vi "Read SerDes GPIO Bank.vi"(0 "verify serdes id":bool=TRUE, 2 "serdes id":T1=enum."SI 0 Deserializer") -> (4 "gpio bank input":T2, 6 "serdes id valid":bool)   [LabVIEW 2023, in "GettingStarted_Common_148X_FPGA.lvlib"]
uses:
  GettingStarted_Common_148X_FPGA.lvlib
  <instrlib>/FlexRIO/CSI-2/v2/FPGA/Types/GPIO Bank.ctl
  Types/SerDes Identifier.ctl
  <instrlib>/_niInstr/Basic Elements/v1/FPGA/niInstr Basic Elements v1 FPGA.lvlib
  <vilib>/eio/EIONode/EIONode.xnode
  <vilib>/rvi/eio/common/nirviEmuTemplateMethod_errors.vi
  <instrlib>/FlexRIO/CSI-2/v2/FPGA/NI CSI-2 API FPGA v2.lvlib
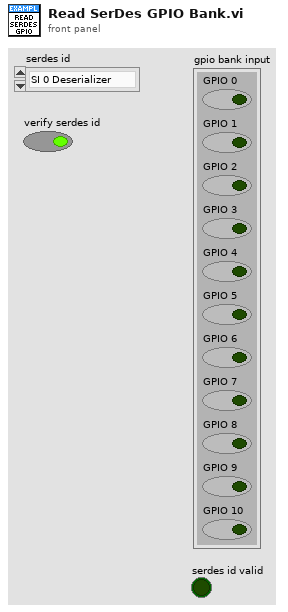
[diagram p1: front panel]
types:
  T1 = typedef "GettingStarted_Common_148X_FPGA.lvlib/SerDes Identifier.ctl" = enum8{"None", "SI 0 Deserializer", "SI 1 Deserializer", "SI 2 Deserializer", "SI 3 Deserializer", "SI 4 Deserializer", "SI 5 Deserializer", "SI 6 Deserializer", "SI 7 Deserializer", "SO 0 Serializer", "SO 1 Serializer", "SO 2 Serializer", "SO 3 Serializer", "SO 4 Serializer", "SO 5 Serializer", "SO 6 Serializer", "SO 7 Serializer", "SI 0 SI 1 Deserializer", "SI 2 SI 3 Deserializer", "SI 4 SI 5 Deserializer", "SI 6 SI 7 Deserializer"}
  T2 = typedef "NI CSI-2 API FPGA v2.lvlib/GPIO Bank.ctl" = cluster{"GPIO 0":bool, "GPIO 1":bool, "GPIO 2":bool, "GPIO 3":bool, "GPIO 4":bool, "GPIO 5":bool, "GPIO 6":bool, "GPIO 7":bool, "GPIO 8":bool, "GPIO 9":bool, "GPIO 10":bool}
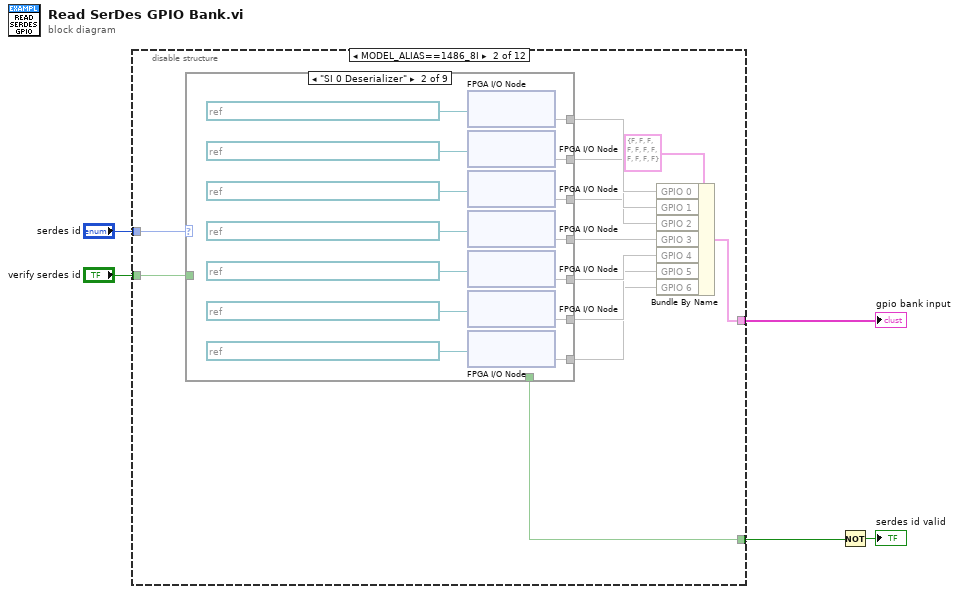
[diagram p0: block diagram]
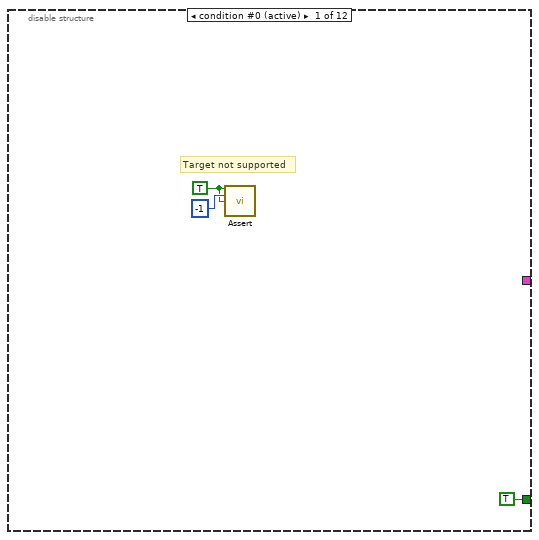
[diagram p2: hidden frame]
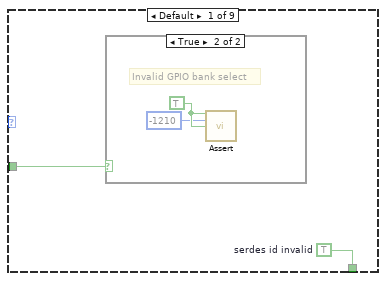
[diagram p3: hidden frame]
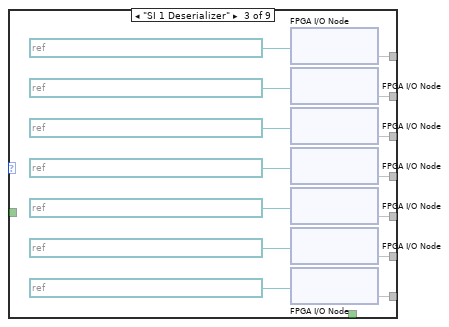
[diagram p5: hidden frame]
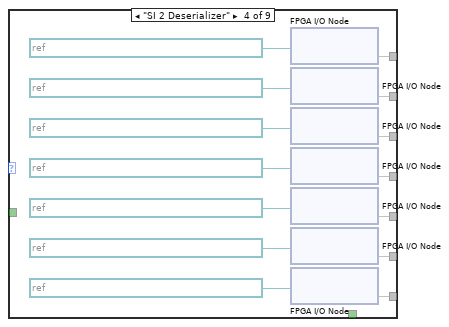
[diagram p6: hidden frame]
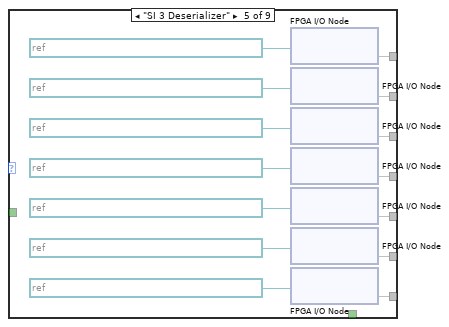
[diagram p7: hidden frame]
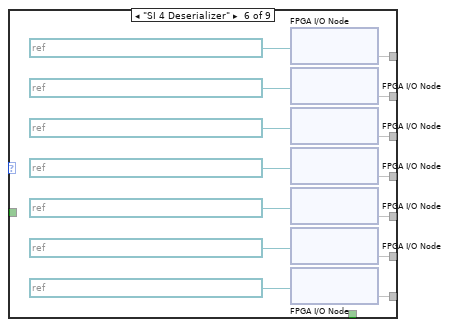
[diagram p8: hidden frame]
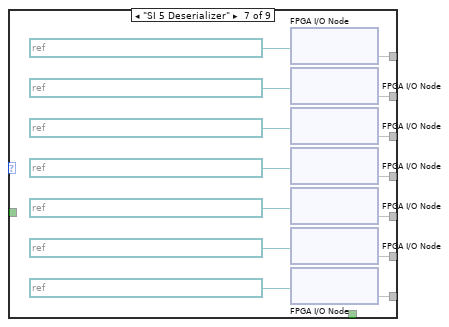
[diagram p9: hidden frame]
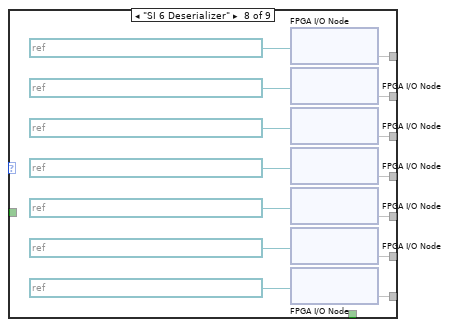
[diagram p10: hidden frame]
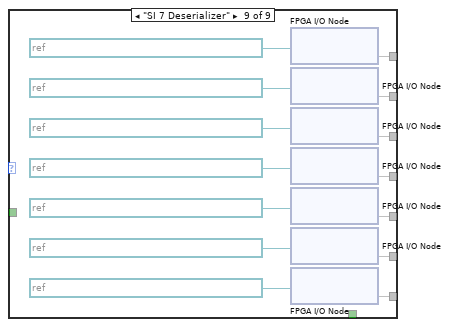
[diagram p11: hidden frame]
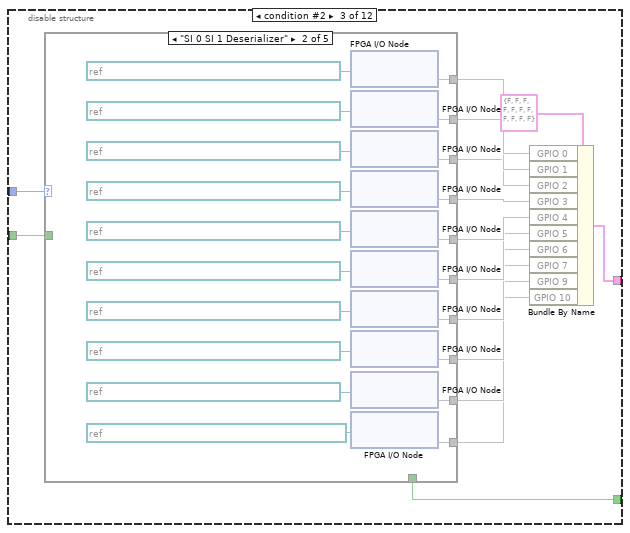
[diagram p12: hidden frame]
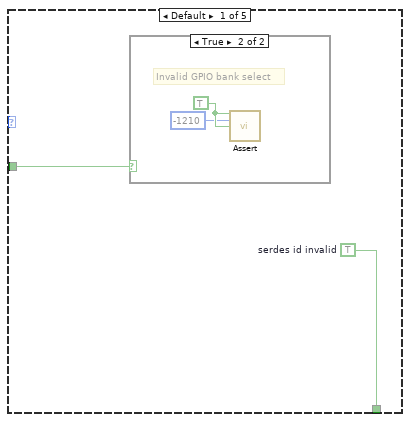
[diagram p13: hidden frame]
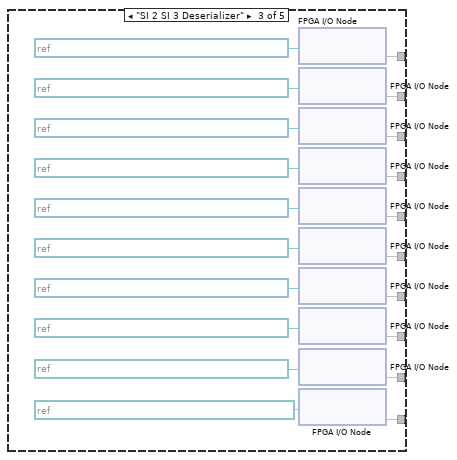
[diagram p15: hidden frame]
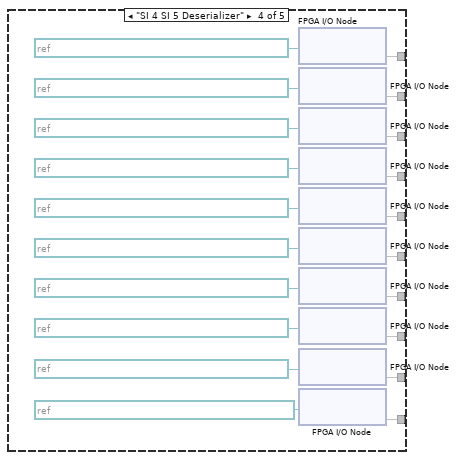
[diagram p16: hidden frame]
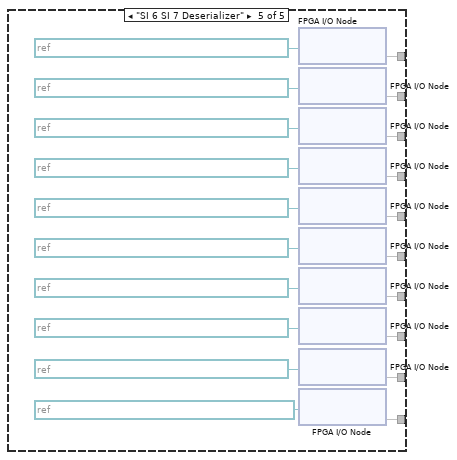
[diagram p17: hidden frame]
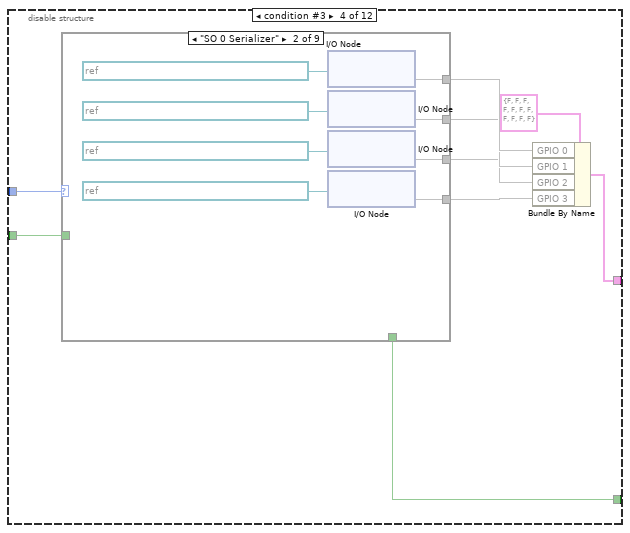
[diagram p18: hidden frame]
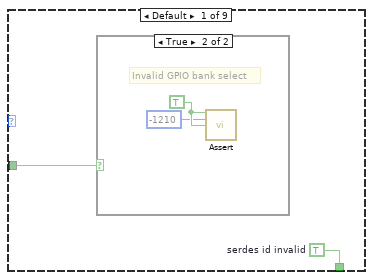
[diagram p19: hidden frame]
diagram:
  n1 = disable-structure shown="MODEL_ALIAS==1486_8I" {
    disable-tunnel: [_ w12 w143 w239 w316 w423 w556 w664 w725 w870 w953 w1125] -> w5
    disable-tunnel: "serdes id" -> [_ w11 w142 w238 w315 w422 w555 w663 w724 w869 w952 w1124]
    disable-tunnel: "verify serdes id" -> [_ w10 w141 w237 w314 w421 w549 w657 w721 w866 w949 w1121]
    disable-tunnel: [TRUE ("serdes gpio bank input select valid") w9 w140 w236 w313 w420 w548 w656 w720 w865 w948 w1120] -> w2
    frame condition #0 (active) {
      w7 = TRUE ("assert")
      # "Target not supported"
      n2 = call <instrlib>:"Assert.vi"("assert"=w7, "error code"=-1, "enable show error"=w7) -> ()  [unwired: 13 in]
    }
    frame condition #1 {
      n3 = case shown="\"SI 0 Deserializer\"" w11 {
        tunnel: [_ w32 w46 w60 w74 w88 w102 w116 w130] -> w19
        tunnel: [_ w31 w45 w59 w73 w87 w101 w115 w129] -> w18
        tunnel: [_ w30 w44 w58 w72 w86 w100 w114 w128] -> w17
        tunnel: [_ w29 w43 w57 w71 w85 w99 w113 w127] -> w16
        tunnel: [_ w28 w42 w56 w70 w84 w98 w112 w126] -> w15
        tunnel: [_ w27 w41 w55 w69 w83 w97 w111 w125] -> w14
        tunnel: [_ w25 w39 w53 w67 w81 w95 w109 w123] -> w13
        tunnel: w10 -> [w22 _ _ _ _ _ _ _ _]
        tunnel: [w21 _ _ _ _ _ _ _ _] -> w9
        frame Default {
          w21 = TRUE  # serdes id invalid
          n4 = case shown="True" w22 {
            frame False {
            }
            frame True {
              w24 = TRUE ("enable show error")
              # "Invalid GPIO bank select"
              n5 = call <instrlib>:"Assert.vi"("assert"=w24, "error code"=-1210, "enable show error"=w24) -> ()  [unwired: 13 in]
            }
          }
        }
        frame "SI 0 Deserializer" {
          n6 = xnode "FPGA I/O Node"("FPGA I/O In"=refnum<k21> "IO Socket\\SI 0 Deserializer GPIO 0 Input") -> ("I/O Item"=w32)  [unwired: 1 out]
          n7 = xnode "FPGA I/O Node"("FPGA I/O In"=refnum<k21> "IO Socket\\SI 0 Deserializer GPIO 1 Input") -> ("I/O Item"=w31)  [unwired: 1 out]
          n8 = xnode "FPGA I/O Node"("FPGA I/O In"=refnum<k21> "IO Socket\\SI 0 Deserializer GPIO 2 Input") -> ("I/O Item"=w30)  [unwired: 1 out]
          n9 = xnode "FPGA I/O Node"("FPGA I/O In"=refnum<k21> "IO Socket\\SI 0 Deserializer GPIO 3 Input") -> ("I/O Item"=w29)  [unwired: 1 out]
          n10 = xnode "FPGA I/O Node"("FPGA I/O In"=refnum<k21> "IO Socket\\SI 0 Deserializer GPIO 4 Input") -> ("I/O Item"=w28)  [unwired: 1 out]
          n11 = xnode "FPGA I/O Node"("FPGA I/O In"=refnum<k21> "IO Socket\\SI 0 Deserializer GPIO 5 Input") -> ("I/O Item"=w27)  [unwired: 1 out]
          n12 = xnode "FPGA I/O Node"("FPGA I/O In"=refnum<k21> "IO Socket\\SI 0 Deserializer GPIO 6 Input") -> ("I/O Item"=w25)  [unwired: 1 out]
        }
        frame "SI 1 Deserializer" {
          n13 = xnode "FPGA I/O Node"("FPGA I/O In"=refnum<k21> "IO Socket\\SI 1 Deserializer GPIO 0 Input") -> ("I/O Item"=w46)  [unwired: 1 out]
          n14 = xnode "FPGA I/O Node"("FPGA I/O In"=refnum<k21> "IO Socket\\SI 1 Deserializer GPIO 1 Input") -> ("I/O Item"=w45)  [unwired: 1 out]
          n15 = xnode "FPGA I/O Node"("FPGA I/O In"=refnum<k21> "IO Socket\\SI 1 Deserializer GPIO 2 Input") -> ("I/O Item"=w44)  [unwired: 1 out]
          n16 = xnode "FPGA I/O Node"("FPGA I/O In"=refnum<k21> "IO Socket\\SI 1 Deserializer GPIO 3 Input") -> ("I/O Item"=w43)  [unwired: 1 out]
          n17 = xnode "FPGA I/O Node"("FPGA I/O In"=refnum<k21> "IO Socket\\SI 1 Deserializer GPIO 4 Input") -> ("I/O Item"=w42)  [unwired: 1 out]
          n18 = xnode "FPGA I/O Node"("FPGA I/O In"=refnum<k21> "IO Socket\\SI 1 Deserializer GPIO 5 Input") -> ("I/O Item"=w41)  [unwired: 1 out]
          n19 = xnode "FPGA I/O Node"("FPGA I/O In"=refnum<k21> "IO Socket\\SI 1 Deserializer GPIO 6 Input") -> ("I/O Item"=w39)  [unwired: 1 out]
        }
        frame "SI 2 Deserializer" {
          n20 = xnode "FPGA I/O Node"("FPGA I/O In"=refnum<k21> "IO Socket\\SI 2 Deserializer GPIO 0 Input") -> ("I/O Item"=w60)  [unwired: 1 out]
          n21 = xnode "FPGA I/O Node"("FPGA I/O In"=refnum<k21> "IO Socket\\SI 2 Deserializer GPIO 1 Input") -> ("I/O Item"=w59)  [unwired: 1 out]
          n22 = xnode "FPGA I/O Node"("FPGA I/O In"=refnum<k21> "IO Socket\\SI 2 Deserializer GPIO 2 Input") -> ("I/O Item"=w58)  [unwired: 1 out]
          n23 = xnode "FPGA I/O Node"("FPGA I/O In"=refnum<k21> "IO Socket\\SI 2 Deserializer GPIO 3 Input") -> ("I/O Item"=w57)  [unwired: 1 out]
          n24 = xnode "FPGA I/O Node"("FPGA I/O In"=refnum<k21> "IO Socket\\SI 2 Deserializer GPIO 4 Input") -> ("I/O Item"=w56)  [unwired: 1 out]
          n25 = xnode "FPGA I/O Node"("FPGA I/O In"=refnum<k21> "IO Socket\\SI 2 Deserializer GPIO 5 Input") -> ("I/O Item"=w55)  [unwired: 1 out]
          n26 = xnode "FPGA I/O Node"("FPGA I/O In"=refnum<k21> "IO Socket\\SI 2 Deserializer GPIO 6 Input") -> ("I/O Item"=w53)  [unwired: 1 out]
        }
        frame "SI 3 Deserializer" {
          n27 = xnode "FPGA I/O Node"("FPGA I/O In"=refnum<k21> "IO Socket\\SI 3 Deserializer GPIO 0 Input") -> ("I/O Item"=w74)  [unwired: 1 out]
          n28 = xnode "FPGA I/O Node"("FPGA I/O In"=refnum<k21> "IO Socket\\SI 3 Deserializer GPIO 1 Input") -> ("I/O Item"=w73)  [unwired: 1 out]
          n29 = xnode "FPGA I/O Node"("FPGA I/O In"=refnum<k21> "IO Socket\\SI 3 Deserializer GPIO 2 Input") -> ("I/O Item"=w72)  [unwired: 1 out]
          n30 = xnode "FPGA I/O Node"("FPGA I/O In"=refnum<k21> "IO Socket\\SI 3 Deserializer GPIO 3 Input") -> ("I/O Item"=w71)  [unwired: 1 out]
          n31 = xnode "FPGA I/O Node"("FPGA I/O In"=refnum<k21> "IO Socket\\SI 3 Deserializer GPIO 4 Input") -> ("I/O Item"=w70)  [unwired: 1 out]
          n32 = xnode "FPGA I/O Node"("FPGA I/O In"=refnum<k21> "IO Socket\\SI 3 Deserializer GPIO 5 Input") -> ("I/O Item"=w69)  [unwired: 1 out]
          n33 = xnode "FPGA I/O Node"("FPGA I/O In"=refnum<k21> "IO Socket\\SI 3 Deserializer GPIO 6 Input") -> ("I/O Item"=w67)  [unwired: 1 out]
        }
        frame "SI 4 Deserializer" {
          n34 = xnode "FPGA I/O Node"("FPGA I/O In"=refnum<k21> "IO Socket\\SI 4 Deserializer GPIO 0 Input") -> ("I/O Item"=w88)  [unwired: 1 out]
          n35 = xnode "FPGA I/O Node"("FPGA I/O In"=refnum<k21> "IO Socket\\SI 4 Deserializer GPIO 1 Input") -> ("I/O Item"=w87)  [unwired: 1 out]
          n36 = xnode "FPGA I/O Node"("FPGA I/O In"=refnum<k21> "IO Socket\\SI 4 Deserializer GPIO 2 Input") -> ("I/O Item"=w86)  [unwired: 1 out]
          n37 = xnode "FPGA I/O Node"("FPGA I/O In"=refnum<k21> "IO Socket\\SI 4 Deserializer GPIO 3 Input") -> ("I/O Item"=w85)  [unwired: 1 out]
          n38 = xnode "FPGA I/O Node"("FPGA I/O In"=refnum<k21> "IO Socket\\SI 4 Deserializer GPIO 4 Input") -> ("I/O Item"=w84)  [unwired: 1 out]
          n39 = xnode "FPGA I/O Node"("FPGA I/O In"=refnum<k21> "IO Socket\\SI 4 Deserializer GPIO 5 Input") -> ("I/O Item"=w83)  [unwired: 1 out]
          n40 = xnode "FPGA I/O Node"("FPGA I/O In"=refnum<k21> "IO Socket\\SI 4 Deserializer GPIO 6 Input") -> ("I/O Item"=w81)  [unwired: 1 out]
        }
        frame "SI 5 Deserializer" {
          n41 = xnode "FPGA I/O Node"("FPGA I/O In"=refnum<k21> "IO Socket\\SI 5 Deserializer GPIO 0 Input") -> ("I/O Item"=w102)  [unwired: 1 out]
          n42 = xnode "FPGA I/O Node"("FPGA I/O In"=refnum<k21> "IO Socket\\SI 5 Deserializer GPIO 1 Input") -> ("I/O Item"=w101)  [unwired: 1 out]
          n43 = xnode "FPGA I/O Node"("FPGA I/O In"=refnum<k21> "IO Socket\\SI 5 Deserializer GPIO 2 Input") -> ("I/O Item"=w100)  [unwired: 1 out]
          n44 = xnode "FPGA I/O Node"("FPGA I/O In"=refnum<k21> "IO Socket\\SI 5 Deserializer GPIO 3 Input") -> ("I/O Item"=w99)  [unwired: 1 out]
          n45 = xnode "FPGA I/O Node"("FPGA I/O In"=refnum<k21> "IO Socket\\SI 5 Deserializer GPIO 4 Input") -> ("I/O Item"=w98)  [unwired: 1 out]
          n46 = xnode "FPGA I/O Node"("FPGA I/O In"=refnum<k21> "IO Socket\\SI 5 Deserializer GPIO 5 Input") -> ("I/O Item"=w97)  [unwired: 1 out]
          n47 = xnode "FPGA I/O Node"("FPGA I/O In"=refnum<k21> "IO Socket\\SI 5 Deserializer GPIO 6 Input") -> ("I/O Item"=w95)  [unwired: 1 out]
        }
        frame "SI 6 Deserializer" {
          n48 = xnode "FPGA I/O Node"("FPGA I/O In"=refnum<k21> "IO Socket\\SI 6 Deserializer GPIO 0 Input") -> ("I/O Item"=w116)  [unwired: 1 out]
          n49 = xnode "FPGA I/O Node"("FPGA I/O In"=refnum<k21> "IO Socket\\SI 6 Deserializer GPIO 1 Input") -> ("I/O Item"=w115)  [unwired: 1 out]
          n50 = xnode "FPGA I/O Node"("FPGA I/O In"=refnum<k21> "IO Socket\\SI 6 Deserializer GPIO 2 Input") -> ("I/O Item"=w114)  [unwired: 1 out]
          n51 = xnode "FPGA I/O Node"("FPGA I/O In"=refnum<k21> "IO Socket\\SI 6 Deserializer GPIO 3 Input") -> ("I/O Item"=w113)  [unwired: 1 out]
          n52 = xnode "FPGA I/O Node"("FPGA I/O In"=refnum<k21> "IO Socket\\SI 6 Deserializer GPIO 4 Input") -> ("I/O Item"=w112)  [unwired: 1 out]
          n53 = xnode "FPGA I/O Node"("FPGA I/O In"=refnum<k21> "IO Socket\\SI 6 Deserializer GPIO 5 Input") -> ("I/O Item"=w111)  [unwired: 1 out]
          n54 = xnode "FPGA I/O Node"("FPGA I/O In"=refnum<k21> "IO Socket\\SI 6 Deserializer GPIO 6 Input") -> ("I/O Item"=w109)  [unwired: 1 out]
        }
        frame "SI 7 Deserializer" {
          n55 = xnode "FPGA I/O Node"("FPGA I/O In"=refnum<k21> "IO Socket\\SI 7 Deserializer GPIO 0 Input") -> ("I/O Item"=w130)  [unwired: 1 out]
          n56 = xnode "FPGA I/O Node"("FPGA I/O In"=refnum<k21> "IO Socket\\SI 7 Deserializer GPIO 1 Input") -> ("I/O Item"=w129)  [unwired: 1 out]
          n57 = xnode "FPGA I/O Node"("FPGA I/O In"=refnum<k21> "IO Socket\\SI 7 Deserializer GPIO 2 Input") -> ("I/O Item"=w128)  [unwired: 1 out]
          n58 = xnode "FPGA I/O Node"("FPGA I/O In"=refnum<k21> "IO Socket\\SI 7 Deserializer GPIO 3 Input") -> ("I/O Item"=w127)  [unwired: 1 out]
          n59 = xnode "FPGA I/O Node"("FPGA I/O In"=refnum<k21> "IO Socket\\SI 7 Deserializer GPIO 4 Input") -> ("I/O Item"=w126)  [unwired: 1 out]
          n60 = xnode "FPGA I/O Node"("FPGA I/O In"=refnum<k21> "IO Socket\\SI 7 Deserializer GPIO 5 Input") -> ("I/O Item"=w125)  [unwired: 1 out]
          n61 = xnode "FPGA I/O Node"("FPGA I/O In"=refnum<k21> "IO Socket\\SI 7 Deserializer GPIO 6 Input") -> ("I/O Item"=w123)  [unwired: 1 out]
        }
      }
      n62 = Bundle By Name(cluster=T2 {"GPIO 0"=FALSE, "GPIO 1"=FALSE, "GPIO 2"=FALSE, "GPIO 3"=FALSE, "GPIO 4"=FALSE, "GPIO 5"=FALSE, "GPIO 6"=FALSE, "GPIO 7"=FALSE, "GPIO 8"=FALSE, "GPIO 9"=FALSE, "GPIO 10"=FALSE} ("gpio bank"), "GPIO 0"=w19, "GPIO 1"=w18, "GPIO 2"=w17, "GPIO 3"=w16, "GPIO 4"=w15, "GPIO 5"=w14, "GPIO 6"=w13) -> (w12:T2)
    }
    frame condition #2 {
      n63 = case shown="\"SI 0 SI 1 Deserializer\"" w142 {
        tunnel: [_ w173 w193 w213 w233] -> w150
        tunnel: [_ w172 w192 w212 w232] -> w149
        tunnel: [_ w171 w191 w211 w231] -> w148
        tunnel: [_ w170 w190 w210 w230] -> w147
        tunnel: [_ w169 w189 w209 w229] -> w146
        tunnel: [_ w168 w188 w208 w228] -> w145
        tunnel: [_ w167 w187 w207 w227] -> w144
        tunnel: w141 -> [w153 _ _ _ _]
        tunnel: [w152 _ _ _ _] -> w140
        tunnel: [_ w165 w185 w205 w225] -> w139
        tunnel: [_ w156 w176 w196 w216] -> w138
        tunnel: [_ w157 w177 w197 w217] -> w137
        frame Default {
          w152 = TRUE  # serdes id invalid
          n64 = case shown="True" w153 {
            frame False {
            }
            frame True {
              w155 = TRUE ("enable show error")
              # "Invalid GPIO bank select"
              n65 = call <instrlib>:"Assert.vi"("assert"=w155, "error code"=-1210, "enable show error"=w155) -> ()  [unwired: 13 in]
            }
          }
        }
        frame "SI 0 SI 1 Deserializer" {
          n66 = xnode "FPGA I/O Node"("FPGA I/O In"=refnum<k21> "IO Socket\\SI 0 SI 1 Deserializer GPIO 0 Input") -> ("I/O Item"=w173)  [unwired: 1 out]
          n67 = xnode "FPGA I/O Node"("FPGA I/O In"=refnum<k21> "IO Socket\\SI 0 SI 1 Deserializer GPIO 1 Input") -> ("I/O Item"=w172)  [unwired: 1 out]
          n68 = xnode "FPGA I/O Node"("FPGA I/O In"=refnum<k21> "IO Socket\\SI 0 SI 1 Deserializer GPIO 2 Input") -> ("I/O Item"=w171)  [unwired: 1 out]
          n69 = xnode "FPGA I/O Node"("FPGA I/O In"=refnum<k21> "IO Socket\\SI 0 SI 1 Deserializer GPIO 3 Input") -> ("I/O Item"=w170)  [unwired: 1 out]
          n70 = xnode "FPGA I/O Node"("FPGA I/O In"=refnum<k21> "IO Socket\\SI 0 SI 1 Deserializer GPIO 4 Input") -> ("I/O Item"=w169)  [unwired: 1 out]
          n71 = xnode "FPGA I/O Node"("FPGA I/O In"=refnum<k21> "IO Socket\\SI 0 SI 1 Deserializer GPIO 5 Input") -> ("I/O Item"=w168)  [unwired: 1 out]
          n72 = xnode "FPGA I/O Node"("FPGA I/O In"=refnum<k21> "IO Socket\\SI 0 SI 1 Deserializer GPIO 6 Input") -> ("I/O Item"=w167)  [unwired: 1 out]
          n73 = xnode "FPGA I/O Node"("FPGA I/O In"=refnum<k21> "IO Socket\\SI 0 SI 1 Deserializer GPIO 7 Input") -> ("I/O Item"=w165)  [unwired: 1 out]
          n74 = xnode "FPGA I/O Node"("FPGA I/O In"=refnum<k21> "IO Socket\\SI 0 SI 1 Deserializer GPIO 9 Input") -> ("I/O Item"=w156)  [unwired: 1 out]
          n75 = xnode "FPGA I/O Node"("FPGA I/O In"=refnum<k21> "IO Socket\\SI 0 SI 1 Deserializer GPIO 10 Input") -> ("I/O Item"=w157)  [unwired: 1 out]
        }
        frame "SI 2 SI 3 Deserializer" {
          n76 = xnode "FPGA I/O Node"("FPGA I/O In"=refnum<k21> "IO Socket\\SI 2 SI 3 Deserializer GPIO 0 Input") -> ("I/O Item"=w193)  [unwired: 1 out]
          n77 = xnode "FPGA I/O Node"("FPGA I/O In"=refnum<k21> "IO Socket\\SI 2 SI 3 Deserializer GPIO 1 Input") -> ("I/O Item"=w192)  [unwired: 1 out]
          n78 = xnode "FPGA I/O Node"("FPGA I/O In"=refnum<k21> "IO Socket\\SI 2 SI 3 Deserializer GPIO 2 Input") -> ("I/O Item"=w191)  [unwired: 1 out]
          n79 = xnode "FPGA I/O Node"("FPGA I/O In"=refnum<k21> "IO Socket\\SI 2 SI 3 Deserializer GPIO 3 Input") -> ("I/O Item"=w190)  [unwired: 1 out]
          n80 = xnode "FPGA I/O Node"("FPGA I/O In"=refnum<k21> "IO Socket\\SI 2 SI 3 Deserializer GPIO 4 Input") -> ("I/O Item"=w189)  [unwired: 1 out]
          n81 = xnode "FPGA I/O Node"("FPGA I/O In"=refnum<k21> "IO Socket\\SI 2 SI 3 Deserializer GPIO 5 Input") -> ("I/O Item"=w188)  [unwired: 1 out]
          n82 = xnode "FPGA I/O Node"("FPGA I/O In"=refnum<k21> "IO Socket\\SI 2 SI 3 Deserializer GPIO 6 Input") -> ("I/O Item"=w187)  [unwired: 1 out]
          n83 = xnode "FPGA I/O Node"("FPGA I/O In"=refnum<k21> "IO Socket\\SI 2 SI 3 Deserializer GPIO 7 Input") -> ("I/O Item"=w185)  [unwired: 1 out]
          n84 = xnode "FPGA I/O Node"("FPGA I/O In"=refnum<k21> "IO Socket\\SI 2 SI 3 Deserializer GPIO 9 Input") -> ("I/O Item"=w176)  [unwired: 1 out]
          n85 = xnode "FPGA I/O Node"("FPGA I/O In"=refnum<k21> "IO Socket\\SI 2 SI 3 Deserializer GPIO 10 Input") -> ("I/O Item"=w177)  [unwired: 1 out]
        }
        frame "SI 4 SI 5 Deserializer" {
          n86 = xnode "FPGA I/O Node"("FPGA I/O In"=refnum<k21> "IO Socket\\SI 4 SI 5 Deserializer GPIO 0 Input") -> ("I/O Item"=w213)  [unwired: 1 out]
          n87 = xnode "FPGA I/O Node"("FPGA I/O In"=refnum<k21> "IO Socket\\SI 4 SI 5 Deserializer GPIO 1 Input") -> ("I/O Item"=w212)  [unwired: 1 out]
          n88 = xnode "FPGA I/O Node"("FPGA I/O In"=refnum<k21> "IO Socket\\SI 4 SI 5 Deserializer GPIO 2 Input") -> ("I/O Item"=w211)  [unwired: 1 out]
          n89 = xnode "FPGA I/O Node"("FPGA I/O In"=refnum<k21> "IO Socket\\SI 4 SI 5 Deserializer GPIO 3 Input") -> ("I/O Item"=w210)  [unwired: 1 out]
          n90 = xnode "FPGA I/O Node"("FPGA I/O In"=refnum<k21> "IO Socket\\SI 4 SI 5 Deserializer GPIO 4 Input") -> ("I/O Item"=w209)  [unwired: 1 out]
          n91 = xnode "FPGA I/O Node"("FPGA I/O In"=refnum<k21> "IO Socket\\SI 4 SI 5 Deserializer GPIO 5 Input") -> ("I/O Item"=w208)  [unwired: 1 out]
          n92 = xnode "FPGA I/O Node"("FPGA I/O In"=refnum<k21> "IO Socket\\SI 4 SI 5 Deserializer GPIO 6 Input") -> ("I/O Item"=w207)  [unwired: 1 out]
          n93 = xnode "FPGA I/O Node"("FPGA I/O In"=refnum<k21> "IO Socket\\SI 4 SI 5 Deserializer GPIO 7 Input") -> ("I/O Item"=w205)  [unwired: 1 out]
          n94 = xnode "FPGA I/O Node"("FPGA I/O In"=refnum<k21> "IO Socket\\SI 4 SI 5 Deserializer GPIO 9 Input") -> ("I/O Item"=w196)  [unwired: 1 out]
          n95 = xnode "FPGA I/O Node"("FPGA I/O In"=refnum<k21> "IO Socket\\SI 4 SI 5 Deserializer GPIO 10 Input") -> ("I/O Item"=w197)  [unwired: 1 out]
        }
        frame "SI 6 SI 7 Deserializer" {
          n96 = xnode "FPGA I/O Node"("FPGA I/O In"=refnum<k21> "IO Socket\\SI 6 SI 7 Deserializer GPIO 0 Input") -> ("I/O Item"=w233)  [unwired: 1 out]
          n97 = xnode "FPGA I/O Node"("FPGA I/O In"=refnum<k21> "IO Socket\\SI 6 SI 7 Deserializer GPIO 1 Input") -> ("I/O Item"=w232)  [unwired: 1 out]
          n98 = xnode "FPGA I/O Node"("FPGA I/O In"=refnum<k21> "IO Socket\\SI 6 SI 7 Deserializer GPIO 2 Input") -> ("I/O Item"=w231)  [unwired: 1 out]
          n99 = xnode "FPGA I/O Node"("FPGA I/O In"=refnum<k21> "IO Socket\\SI 6 SI 7 Deserializer GPIO 3 Input") -> ("I/O Item"=w230)  [unwired: 1 out]
          n100 = xnode "FPGA I/O Node"("FPGA I/O In"=refnum<k21> "IO Socket\\SI 6 SI 7 Deserializer GPIO 4 Input") -> ("I/O Item"=w229)  [unwired: 1 out]
          n101 = xnode "FPGA I/O Node"("FPGA I/O In"=refnum<k21> "IO Socket\\SI 6 SI 7 Deserializer GPIO 5 Input") -> ("I/O Item"=w228)  [unwired: 1 out]
          n102 = xnode "FPGA I/O Node"("FPGA I/O In"=refnum<k21> "IO Socket\\SI 6 SI 7 Deserializer GPIO 6 Input") -> ("I/O Item"=w227)  [unwired: 1 out]
          n103 = xnode "FPGA I/O Node"("FPGA I/O In"=refnum<k21> "IO Socket\\SI 6 SI 7 Deserializer GPIO 7 Input") -> ("I/O Item"=w225)  [unwired: 1 out]
          n104 = xnode "FPGA I/O Node"("FPGA I/O In"=refnum<k21> "IO Socket\\SI 6 SI 7 Deserializer GPIO 9 Input") -> ("I/O Item"=w216)  [unwired: 1 out]
          n105 = xnode "FPGA I/O Node"("FPGA I/O In"=refnum<k21> "IO Socket\\SI 6 SI 7 Deserializer GPIO 10 Input") -> ("I/O Item"=w217)  [unwired: 1 out]
        }
      }
      n106 = Bundle By Name(cluster=T2 {"GPIO 0"=FALSE, "GPIO 1"=FALSE, "GPIO 2"=FALSE, "GPIO 3"=FALSE, "GPIO 4"=FALSE, "GPIO 5"=FALSE, "GPIO 6"=FALSE, "GPIO 7"=FALSE, "GPIO 8"=FALSE, "GPIO 9"=FALSE, "GPIO 10"=FALSE} ("gpio bank"), "GPIO 0"=w150, "GPIO 1"=w149, "GPIO 2"=w148, "GPIO 3"=w147, "GPIO 4"=w146, "GPIO 5"=w145, "GPIO 6"=w144, "GPIO 7"=w139, "GPIO 9"=w138, "GPIO 10"=w137) -> (w143:T2)
    }
    frame condition #3 {
      n107 = case shown="\"SO 0 Serializer\"" w238 {
        tunnel: [_ w252 w260 w268 w276 w284 w292 w300 w308] -> w243
        tunnel: [_ w251 w259 w267 w275 w283 w291 w299 w307] -> w242
        tunnel: [_ w250 w258 w266 w274 w282 w290 w298 w306] -> w241
        tunnel: [_ w249 w257 w265 w273 w281 w289 w297 w305] -> w240
        tunnel: w237 -> [w246 _ _ _ _ _ _ _ _]
        tunnel: [w245 _ _ _ _ _ _ _ _] -> w236
        frame Default {
          w245 = TRUE  # serdes id invalid
          n108 = case shown="True" w246 {
            frame False {
            }
            frame True {
              w248 = TRUE ("enable show error")
              # "Invalid GPIO bank select"
              n109 = call <instrlib>:"Assert.vi"("assert"=w248, "error code"=-1210, "enable show error"=w248) -> ()  [unwired: 13 in]
            }
          }
        }
        frame "SO 0 Serializer" {
          n110 = xnode "I/O Node"("FPGA I/O In"=refnum<k21> "IO Socket\\SO 0 Serializer GPIO 0 Input") -> ("I/O Item"=w252)  [unwired: 1 out]
          n111 = xnode "I/O Node"("FPGA I/O In"=refnum<k21> "IO Socket\\SO 0 Serializer GPIO 1 Input") -> ("I/O Item"=w251)  [unwired: 1 out]
          n112 = xnode "I/O Node"("FPGA I/O In"=refnum<k21> "IO Socket\\SO 0 Serializer GPIO 2 Input") -> ("I/O Item"=w250)  [unwired: 1 out]
          n113 = xnode "I/O Node"("FPGA I/O In"=refnum<k21> "IO Socket\\SO 0 Serializer GPIO 3 Input") -> ("I/O Item"=w249)  [unwired: 1 out]
        }
        frame "SO 1 Serializer" {
          n114 = xnode "I/O Node"("FPGA I/O In"=refnum<k21> "IO Socket\\SO 1 Serializer GPIO 0 Input") -> ("I/O Item"=w260)  [unwired: 1 out]
          n115 = xnode "I/O Node"("FPGA I/O In"=refnum<k21> "IO Socket\\SO 1 Serializer GPIO 1 Input") -> ("I/O Item"=w259)  [unwired: 1 out]
          n116 = xnode "I/O Node"("FPGA I/O In"=refnum<k21> "IO Socket\\SO 1 Serializer GPIO 2 Input") -> ("I/O Item"=w258)  [unwired: 1 out]
          n117 = xnode "I/O Node"("FPGA I/O In"=refnum<k21> "IO Socket\\SO 1 Serializer GPIO 3 Input") -> ("I/O Item"=w257)  [unwired: 1 out]
        }
        frame "SO 2 Serializer" {
          n118 = xnode "I/O Node"("FPGA I/O In"=refnum<k21> "IO Socket\\SO 2 Serializer GPIO 0 Input") -> ("I/O Item"=w268)  [unwired: 1 out]
          n119 = xnode "I/O Node"("FPGA I/O In"=refnum<k21> "IO Socket\\SO 2 Serializer GPIO 1 Input") -> ("I/O Item"=w267)  [unwired: 1 out]
          n120 = xnode "I/O Node"("FPGA I/O In"=refnum<k21> "IO Socket\\SO 2 Serializer GPIO 2 Input") -> ("I/O Item"=w266)  [unwired: 1 out]
          n121 = xnode "I/O Node"("FPGA I/O In"=refnum<k21> "IO Socket\\SO 2 Serializer GPIO 3 Input") -> ("I/O Item"=w265)  [unwired: 1 out]
        }
        frame "SO 3 Serializer" {
          n122 = xnode "I/O Node"("FPGA I/O In"=refnum<k21> "IO Socket\\SO 3 Serializer GPIO 0 Input") -> ("I/O Item"=w276)  [unwired: 1 out]
          n123 = xnode "I/O Node"("FPGA I/O In"=refnum<k21> "IO Socket\\SO 3 Serializer GPIO 1 Input") -> ("I/O Item"=w275)  [unwired: 1 out]
          n124 = xnode "FPGA I/O Node"("FPGA I/O In"=refnum<k21> "IO Socket\\SO 3 Serializer GPIO 2 Input") -> ("I/O Item"=w274)  [unwired: 1 out]
          n125 = xnode "I/O Node"("FPGA I/O In"=refnum<k21> "IO Socket\\SO 3 Serializer GPIO 3 Input") -> ("I/O Item"=w273)  [unwired: 1 out]
        }
        frame "SO 4 Serializer" {
          n126 = xnode "I/O Node"("FPGA I/O In"=refnum<k21> "IO Socket\\SO 4 Serializer GPIO 0 Input") -> ("I/O Item"=w284)  [unwired: 1 out]
          n127 = xnode "I/O Node"("FPGA I/O In"=refnum<k21> "IO Socket\\SO 4 Serializer GPIO 1 Input") -> ("I/O Item"=w283)  [unwired: 1 out]
          n128 = xnode "I/O Node"("FPGA I/O In"=refnum<k21> "IO Socket\\SO 4 Serializer GPIO 2 Input") -> ("I/O Item"=w282)  [unwired: 1 out]
          n129 = xnode "I/O Node"("FPGA I/O In"=refnum<k21> "IO Socket\\SO 4 Serializer GPIO 3 Input") -> ("I/O Item"=w281)  [unwired: 1 out]
        }
        frame "SO 5 Serializer" {
          n130 = xnode "I/O Node"("FPGA I/O In"=refnum<k21> "IO Socket\\SO 5 Serializer GPIO 0 Input") -> ("I/O Item"=w292)  [unwired: 1 out]
          n131 = xnode "I/O Node"("FPGA I/O In"=refnum<k21> "IO Socket\\SO 5 Serializer GPIO 1 Input") -> ("I/O Item"=w291)  [unwired: 1 out]
          n132 = xnode "I/O Node"("FPGA I/O In"=refnum<k21> "IO Socket\\SO 5 Serializer GPIO 2 Input") -> ("I/O Item"=w290)  [unwired: 1 out]
          n133 = xnode "I/O Node"("FPGA I/O In"=refnum<k21> "IO Socket\\SO 5 Serializer GPIO 3 Input") -> ("I/O Item"=w289)  [unwired: 1 out]
        }
        frame "SO 6 Serializer" {
          n134 = xnode "I/O Node"("FPGA I/O In"=refnum<k21> "IO Socket\\SO 6 Serializer GPIO 0 Input") -> ("I/O Item"=w300)  [unwired: 1 out]
          n135 = xnode "I/O Node"("FPGA I/O In"=refnum<k21> "IO Socket\\SO 6 Serializer GPIO 1 Input") -> ("I/O Item"=w299)  [unwired: 1 out]
          n136 = xnode "I/O Node"("FPGA I/O In"=refnum<k21> "IO Socket\\SO 6 Serializer GPIO 2 Input") -> ("I/O Item"=w298)  [unwired: 1 out]
          n137 = xnode "I/O Node"("FPGA I/O In"=refnum<k21> "IO Socket\\SO 6 Serializer GPIO 3 Input") -> ("I/O Item"=w297)  [unwired: 1 out]
        }
        frame "SO 7 Serializer" {
          n138 = xnode "I/O Node"("FPGA I/O In"=refnum<k21> "IO Socket\\SO 7 Serializer GPIO 0 Input") -> ("I/O Item"=w308)  [unwired: 1 out]
          n139 = xnode "FPGA I/O Node"("FPGA I/O In"=refnum<k21> "IO Socket\\SO 7 Serializer GPIO 1 Input") -> ("I/O Item"=w307)  [unwired: 1 out]
          n140 = xnode "I/O Node"("FPGA I/O In"=refnum<k21> "IO Socket\\SO 7 Serializer GPIO 2 Input") -> ("I/O Item"=w306)  [unwired: 1 out]
          n141 = xnode "I/O Node"("FPGA I/O In"=refnum<k21> "IO Socket\\SO 7 Serializer GPIO 3 Input") -> ("I/O Item"=w305)  [unwired: 1 out]
        }
      }
      n142 = Bundle By Name(cluster=T2 {"GPIO 0"=FALSE, "GPIO 1"=FALSE, "GPIO 2"=FALSE, "GPIO 3"=FALSE, "GPIO 4"=FALSE, "GPIO 5"=FALSE, "GPIO 6"=FALSE, "GPIO 7"=FALSE, "GPIO 8"=FALSE, "GPIO 9"=FALSE, "GPIO 10"=FALSE} ("gpio bank"), "GPIO 0"=w243, "GPIO 1"=w242, "GPIO 2"=w241, "GPIO 3"=w240) -> (w239:T2)
    }
    frame condition #4 {
      n143 = case shown="\"SI 0 Deserializer\"" w315 {
        tunnel: [_ w336 w350 w364 w378 w388 w396 w404 w412] -> w323
        tunnel: [_ w335 w349 w363 w377 w387 w395 w403 w411] -> w322
        tunnel: [_ w334 w348 w362 w376 w386 w394 w402 w410] -> w321
        tunnel: [_ w333 w347 w361 w375 w385 w393 w401 w409] -> w320
        tunnel: [_ w332 w346 w360 w374 _ _ _ _] -> w319
        tunnel: [_ w331 w345 w359 w373 _ _ _ _] -> w318
        tunnel: [_ w329 w343 w357 w371 _ _ _ _] -> w317
        tunnel: w314 -> [w326 _ _ _ _ _ _ _ _]
        tunnel: [w325 _ _ _ _ _ _ _ _] -> w313
        frame Default {
          w325 = TRUE  # serdes id invalid
          n144 = case shown="True" w326 {
            frame False {
            }
            frame True {
              w328 = TRUE ("enable show error")
              # "Invalid GPIO bank select"
              n145 = call <instrlib>:"Assert.vi"("assert"=w328, "error code"=-1210, "enable show error"=w328) -> ()  [unwired: 13 in]
            }
          }
        }
        frame "SI 0 Deserializer" {
          n146 = xnode "FPGA I/O Node"("FPGA I/O In"=refnum<k21> "IO Socket\\SI 0 Deserializer GPIO 0 Input") -> ("I/O Item"=w336)  [unwired: 1 out]
          n147 = xnode "FPGA I/O Node"("FPGA I/O In"=refnum<k21> "IO Socket\\SI 0 Deserializer GPIO 1 Input") -> ("I/O Item"=w335)  [unwired: 1 out]
          n148 = xnode "FPGA I/O Node"("FPGA I/O In"=refnum<k21> "IO Socket\\SI 0 Deserializer GPIO 2 Input") -> ("I/O Item"=w334)  [unwired: 1 out]
          n149 = xnode "FPGA I/O Node"("FPGA I/O In"=refnum<k21> "IO Socket\\SI 0 Deserializer GPIO 3 Input") -> ("I/O Item"=w333)  [unwired: 1 out]
          n150 = xnode "FPGA I/O Node"("FPGA I/O In"=refnum<k21> "IO Socket\\SI 0 Deserializer GPIO 4 Input") -> ("I/O Item"=w332)  [unwired: 1 out]
          n151 = xnode "FPGA I/O Node"("FPGA I/O In"=refnum<k21> "IO Socket\\SI 0 Deserializer GPIO 5 Input") -> ("I/O Item"=w331)  [unwired: 1 out]
          n152 = xnode "FPGA I/O Node"("FPGA I/O In"=refnum<k21> "IO Socket\\SI 0 Deserializer GPIO 6 Input") -> ("I/O Item"=w329)  [unwired: 1 out]
        }
        frame "SI 1 Deserializer" {
          n153 = xnode "FPGA I/O Node"("FPGA I/O In"=refnum<k21> "IO Socket\\SI 1 Deserializer GPIO 0 Input") -> ("I/O Item"=w350)  [unwired: 1 out]
          n154 = xnode "FPGA I/O Node"("FPGA I/O In"=refnum<k21> "IO Socket\\SI 1 Deserializer GPIO 1 Input") -> ("I/O Item"=w349)  [unwired: 1 out]
          n155 = xnode "FPGA I/O Node"("FPGA I/O In"=refnum<k21> "IO Socket\\SI 1 Deserializer GPIO 2 Input") -> ("I/O Item"=w348)  [unwired: 1 out]
          n156 = xnode "FPGA I/O Node"("FPGA I/O In"=refnum<k21> "IO Socket\\SI 1 Deserializer GPIO 3 Input") -> ("I/O Item"=w347)  [unwired: 1 out]
          n157 = xnode "FPGA I/O Node"("FPGA I/O In"=refnum<k21> "IO Socket\\SI 1 Deserializer GPIO 4 Input") -> ("I/O Item"=w346)  [unwired: 1 out]
          n158 = xnode "FPGA I/O Node"("FPGA I/O In"=refnum<k21> "IO Socket\\SI 1 Deserializer GPIO 5 Input") -> ("I/O Item"=w345)  [unwired: 1 out]
          n159 = xnode "FPGA I/O Node"("FPGA I/O In"=refnum<k21> "IO Socket\\SI 1 Deserializer GPIO 6 Input") -> ("I/O Item"=w343)  [unwired: 1 out]
        }
        frame "SI 2 Deserializer" {
          n160 = xnode "FPGA I/O Node"("FPGA I/O In"=refnum<k21> "IO Socket\\SI 2 Deserializer GPIO 0 Input") -> ("I/O Item"=w364)  [unwired: 1 out]
          n161 = xnode "FPGA I/O Node"("FPGA I/O In"=refnum<k21> "IO Socket\\SI 2 Deserializer GPIO 1 Input") -> ("I/O Item"=w363)  [unwired: 1 out]
          n162 = xnode "FPGA I/O Node"("FPGA I/O In"=refnum<k21> "IO Socket\\SI 2 Deserializer GPIO 2 Input") -> ("I/O Item"=w362)  [unwired: 1 out]
          n163 = xnode "FPGA I/O Node"("FPGA I/O In"=refnum<k21> "IO Socket\\SI 2 Deserializer GPIO 3 Input") -> ("I/O Item"=w361)  [unwired: 1 out]
          n164 = xnode "FPGA I/O Node"("FPGA I/O In"=refnum<k21> "IO Socket\\SI 2 Deserializer GPIO 4 Input") -> ("I/O Item"=w360)  [unwired: 1 out]
          n165 = xnode "FPGA I/O Node"("FPGA I/O In"=refnum<k21> "IO Socket\\SI 2 Deserializer GPIO 5 Input") -> ("I/O Item"=w359)  [unwired: 1 out]
          n166 = xnode "FPGA I/O Node"("FPGA I/O In"=refnum<k21> "IO Socket\\SI 2 Deserializer GPIO 6 Input") -> ("I/O Item"=w357)  [unwired: 1 out]
        }
        frame "SI 3 Deserializer" {
          n167 = xnode "FPGA I/O Node"("FPGA I/O In"=refnum<k21> "IO Socket\\SI 3 Deserializer GPIO 0 Input") -> ("I/O Item"=w378)  [unwired: 1 out]
          n168 = xnode "FPGA I/O Node"("FPGA I/O In"=refnum<k21> "IO Socket\\SI 3 Deserializer GPIO 1 Input") -> ("I/O Item"=w377)  [unwired: 1 out]
          n169 = xnode "FPGA I/O Node"("FPGA I/O In"=refnum<k21> "IO Socket\\SI 3 Deserializer GPIO 2 Input") -> ("I/O Item"=w376)  [unwired: 1 out]
          n170 = xnode "FPGA I/O Node"("FPGA I/O In"=refnum<k21> "IO Socket\\SI 3 Deserializer GPIO 3 Input") -> ("I/O Item"=w375)  [unwired: 1 out]
          n171 = xnode "FPGA I/O Node"("FPGA I/O In"=refnum<k21> "IO Socket\\SI 3 Deserializer GPIO 4 Input") -> ("I/O Item"=w374)  [unwired: 1 out]
          n172 = xnode "FPGA I/O Node"("FPGA I/O In"=refnum<k21> "IO Socket\\SI 3 Deserializer GPIO 5 Input") -> ("I/O Item"=w373)  [unwired: 1 out]
          n173 = xnode "FPGA I/O Node"("FPGA I/O In"=refnum<k21> "IO Socket\\SI 3 Deserializer GPIO 6 Input") -> ("I/O Item"=w371)  [unwired: 1 out]
        }
        frame "SO 0 Serializer" {
          n174 = xnode "FPGA I/O Node"("FPGA I/O In"=refnum<k21> "IO Socket\\SO 0 Serializer GPIO 0 Input") -> ("I/O Item"=w388)  [unwired: 1 out]
          n175 = xnode "FPGA I/O Node"("FPGA I/O In"=refnum<k21> "IO Socket\\SO 0 Serializer GPIO 1 Input") -> ("I/O Item"=w387)  [unwired: 1 out]
          n176 = xnode "FPGA I/O Node"("FPGA I/O In"=refnum<k21> "IO Socket\\SO 0 Serializer GPIO 2 Input") -> ("I/O Item"=w386)  [unwired: 1 out]
          n177 = xnode "FPGA I/O Node"("FPGA I/O In"=refnum<k21> "IO Socket\\SO 0 Serializer GPIO 3 Input") -> ("I/O Item"=w385)  [unwired: 1 out]
        }
        frame "SO 1 Serializer" {
          n178 = xnode "FPGA I/O Node"("FPGA I/O In"=refnum<k21> "IO Socket\\SO 1 Serializer GPIO 0 Input") -> ("I/O Item"=w396)  [unwired: 1 out]
          n179 = xnode "FPGA I/O Node"("FPGA I/O In"=refnum<k21> "IO Socket\\SO 1 Serializer GPIO 1 Input") -> ("I/O Item"=w395)  [unwired: 1 out]
          n180 = xnode "FPGA I/O Node"("FPGA I/O In"=refnum<k21> "IO Socket\\SO 1 Serializer GPIO 2 Input") -> ("I/O Item"=w394)  [unwired: 1 out]
          n181 = xnode "FPGA I/O Node"("FPGA I/O In"=refnum<k21> "IO Socket\\SO 1 Serializer GPIO 3 Input") -> ("I/O Item"=w393)  [unwired: 1 out]
        }
        frame "SO 2 Serializer" {
          n182 = xnode "FPGA I/O Node"("FPGA I/O In"=refnum<k21> "IO Socket\\SO 2 Serializer GPIO 0 Input") -> ("I/O Item"=w404)  [unwired: 1 out]
          n183 = xnode "FPGA I/O Node"("FPGA I/O In"=refnum<k21> "IO Socket\\SO 2 Serializer GPIO 1 Input") -> ("I/O Item"=w403)  [unwired: 1 out]
          n184 = xnode "FPGA I/O Node"("FPGA I/O In"=refnum<k21> "IO Socket\\SO 2 Serializer GPIO 2 Input") -> ("I/O Item"=w402)  [unwired: 1 out]
          n185 = xnode "FPGA I/O Node"("FPGA I/O In"=refnum<k21> "IO Socket\\SO 2 Serializer GPIO 3 Input") -> ("I/O Item"=w401)  [unwired: 1 out]
        }
        frame "SO 3 Serializer" {
          n186 = xnode "FPGA I/O Node"("FPGA I/O In"=refnum<k21> "IO Socket\\SO 3 Serializer GPIO 0 Input") -> ("I/O Item"=w412)  [unwired: 1 out]
          n187 = xnode "FPGA I/O Node"("FPGA I/O In"=refnum<k21> "IO Socket\\SO 3 Serializer GPIO 1 Input") -> ("I/O Item"=w411)  [unwired: 1 out]
          n188 = xnode "FPGA I/O Node"("FPGA I/O In"=refnum<k21> "IO Socket\\SO 3 Serializer GPIO 2 Input") -> ("I/O Item"=w410)  [unwired: 1 out]
          n189 = xnode "FPGA I/O Node"("FPGA I/O In"=refnum<k21> "IO Socket\\SO 3 Serializer GPIO 3 Input") -> ("I/O Item"=w409)  [unwired: 1 out]
        }
      }
      n190 = Bundle By Name(cluster=T2 {"GPIO 0"=FALSE, "GPIO 1"=FALSE, "GPIO 2"=FALSE, "GPIO 3"=FALSE, "GPIO 4"=FALSE, "GPIO 5"=FALSE, "GPIO 6"=FALSE, "GPIO 7"=FALSE, "GPIO 8"=FALSE, "GPIO 9"=FALSE, "GPIO 10"=FALSE} ("gpio bank"), "GPIO 0"=w323, "GPIO 1"=w322, "GPIO 2"=w321, "GPIO 3"=w320, "GPIO 4"=w319, "GPIO 5"=w318, "GPIO 6"=w317) -> (w316:T2)
    }
    frame condition #5 {
      n191 = case shown="\"SI 0 Deserializer\"" w422 {
        tunnel: [_ w449 w469 w489 w509 w519 w527 w535 w543] -> w430
        tunnel: [_ w448 w468 w488 w508 w518 w526 w534 w542] -> w429
        tunnel: [_ w447 w467 w487 w507 w517 w525 w533 w541] -> w428
        tunnel: [_ w446 w466 w486 w506 w516 w524 w532 w540] -> w427
        tunnel: [_ w445 w465 w485 w505 _ _ _ _] -> w426
        tunnel: [_ w444 w464 w484 w504 _ _ _ _] -> w425
        tunnel: [_ w442 w462 w482 w502 _ _ _ _] -> w424
        tunnel: w421 -> [w433 _ _ _ _ _ _ _ _]
        tunnel: [w432 _ _ _ _ _ _ _ _] -> w420
        tunnel: [_ w438 w456 w476 w496 _ _ _ _] -> w419
        tunnel: [_ w437 w459 w477 w497 _ _ _ _] -> w418
        tunnel: [_ w436 w458 w478 w498 _ _ _ _] -> w417
        frame Default {
          w432 = TRUE  # serdes id invalid
          n192 = case shown="False" w433 {
            frame False {
            }
            frame True {
              w435 = TRUE ("enable show error")
              # "Invalid GPIO bank select"
              n193 = call <instrlib>:"Assert.vi"("assert"=w435, "error code"=-1210, "enable show error"=w435) -> ()  [unwired: 13 in]
            }
          }
        }
        frame "SI 0 Deserializer" {
          n194 = xnode "FPGA I/O Node"("FPGA I/O In"=refnum<k21> "IO Socket\\SI 0 Deserializer GPIO 0 Input") -> ("I/O Item"=w449)  [unwired: 1 out]
          n195 = xnode "FPGA I/O Node"("FPGA I/O In"=refnum<k21> "IO Socket\\SI 0 Deserializer GPIO 1 Input") -> ("I/O Item"=w448)  [unwired: 1 out]
          n196 = xnode "FPGA I/O Node"("FPGA I/O In"=refnum<k21> "IO Socket\\SI 0 Deserializer GPIO 2 Input") -> ("I/O Item"=w447)  [unwired: 1 out]
          n197 = xnode "FPGA I/O Node"("FPGA I/O In"=refnum<k21> "IO Socket\\SI 0 Deserializer GPIO 3 Input") -> ("I/O Item"=w446)  [unwired: 1 out]
          n198 = xnode "FPGA I/O Node"("FPGA I/O In"=refnum<k21> "IO Socket\\SI 0 Deserializer GPIO 4 Input") -> ("I/O Item"=w445)  [unwired: 1 out]
          n199 = xnode "FPGA I/O Node"("FPGA I/O In"=refnum<k21> "IO Socket\\SI 0 Deserializer GPIO 5 Input") -> ("I/O Item"=w444)  [unwired: 1 out]
          n200 = xnode "FPGA I/O Node"("FPGA I/O In"=refnum<k21> "IO Socket\\SI 0 Deserializer GPIO 6 Input") -> ("I/O Item"=w442)  [unwired: 1 out]
          n201 = xnode "FPGA I/O Node"("FPGA I/O In"=refnum<k21> "IO Socket\\SI 0 Deserializer GPIO 7 Input") -> ("I/O Item"=w438)  [unwired: 1 out]
          n202 = xnode "FPGA I/O Node"("FPGA I/O In"=refnum<k21> "IO Socket\\SI 0 Deserializer GPIO 9 Input") -> ("I/O Item"=w437)  [unwired: 1 out]
          n203 = xnode "FPGA I/O Node"("FPGA I/O In"=refnum<k21> "IO Socket\\SI 0 Deserializer GPIO 10 Input") -> ("I/O Item"=w436)  [unwired: 1 out]
        }
        frame "SI 1 Deserializer" {
          n204 = xnode "FPGA I/O Node"("FPGA I/O In"=refnum<k21> "IO Socket\\SI 1 Deserializer GPIO 0 Input") -> ("I/O Item"=w469)  [unwired: 1 out]
          n205 = xnode "FPGA I/O Node"("FPGA I/O In"=refnum<k21> "IO Socket\\SI 1 Deserializer GPIO 1 Input") -> ("I/O Item"=w468)  [unwired: 1 out]
          n206 = xnode "FPGA I/O Node"("FPGA I/O In"=refnum<k21> "IO Socket\\SI 1 Deserializer GPIO 2 Input") -> ("I/O Item"=w467)  [unwired: 1 out]
          n207 = xnode "FPGA I/O Node"("FPGA I/O In"=refnum<k21> "IO Socket\\SI 1 Deserializer GPIO 3 Input") -> ("I/O Item"=w466)  [unwired: 1 out]
          n208 = xnode "FPGA I/O Node"("FPGA I/O In"=refnum<k21> "IO Socket\\SI 1 Deserializer GPIO 4 Input") -> ("I/O Item"=w465)  [unwired: 1 out]
          n209 = xnode "FPGA I/O Node"("FPGA I/O In"=refnum<k21> "IO Socket\\SI 1 Deserializer GPIO 5 Input") -> ("I/O Item"=w464)  [unwired: 1 out]
          n210 = xnode "FPGA I/O Node"("FPGA I/O In"=refnum<k21> "IO Socket\\SI 1 Deserializer GPIO 6 Input") -> ("I/O Item"=w462)  [unwired: 1 out]
          n211 = xnode "FPGA I/O Node"("FPGA I/O In"=refnum<k21> "IO Socket\\SI 1 Deserializer GPIO 7 Input") -> ("I/O Item"=w456)  [unwired: 1 out]
          n212 = xnode "FPGA I/O Node"("FPGA I/O In"=refnum<k21> "IO Socket\\SI 1 Deserializer GPIO 9 Input") -> ("I/O Item"=w459)  [unwired: 1 out]
          n213 = xnode "FPGA I/O Node"("FPGA I/O In"=refnum<k21> "IO Socket\\SI 1 Deserializer GPIO 10 Input") -> ("I/O Item"=w458)  [unwired: 1 out]
        }
        frame "SI 2 Deserializer" {
          n214 = xnode "FPGA I/O Node"("FPGA I/O In"=refnum<k21> "IO Socket\\SI 2 Deserializer GPIO 0 Input") -> ("I/O Item"=w489)  [unwired: 1 out]
          n215 = xnode "FPGA I/O Node"("FPGA I/O In"=refnum<k21> "IO Socket\\SI 2 Deserializer GPIO 1 Input") -> ("I/O Item"=w488)  [unwired: 1 out]
          n216 = xnode "FPGA I/O Node"("FPGA I/O In"=refnum<k21> "IO Socket\\SI 2 Deserializer GPIO 2 Input") -> ("I/O Item"=w487)  [unwired: 1 out]
          n217 = xnode "FPGA I/O Node"("FPGA I/O In"=refnum<k21> "IO Socket\\SI 2 Deserializer GPIO 3 Input") -> ("I/O Item"=w486)  [unwired: 1 out]
          n218 = xnode "FPGA I/O Node"("FPGA I/O In"=refnum<k21> "IO Socket\\SI 2 Deserializer GPIO 4 Input") -> ("I/O Item"=w485)  [unwired: 1 out]
          n219 = xnode "FPGA I/O Node"("FPGA I/O In"=refnum<k21> "IO Socket\\SI 2 Deserializer GPIO 5 Input") -> ("I/O Item"=w484)  [unwired: 1 out]
          n220 = xnode "FPGA I/O Node"("FPGA I/O In"=refnum<k21> "IO Socket\\SI 2 Deserializer GPIO 6 Input") -> ("I/O Item"=w482)  [unwired: 1 out]
          n221 = xnode "FPGA I/O Node"("FPGA I/O In"=refnum<k21> "IO Socket\\SI 2 Deserializer GPIO 7 Input") -> ("I/O Item"=w476)  [unwired: 1 out]
          n222 = xnode "FPGA I/O Node"("FPGA I/O In"=refnum<k21> "IO Socket\\SI 2 Deserializer GPIO 9 Input") -> ("I/O Item"=w477)  [unwired: 1 out]
          n223 = xnode "FPGA I/O Node"("FPGA I/O In"=refnum<k21> "IO Socket\\SI 2 Deserializer GPIO 10 Input") -> ("I/O Item"=w478)  [unwired: 1 out]
        }
        frame "SI 3 Deserializer" {
          n224 = xnode "FPGA I/O Node"("FPGA I/O In"=refnum<k21> "IO Socket\\SI 3 Deserializer GPIO 0 Input") -> ("I/O Item"=w509)  [unwired: 1 out]
          n225 = xnode "FPGA I/O Node"("FPGA I/O In"=refnum<k21> "IO Socket\\SI 3 Deserializer GPIO 1 Input") -> ("I/O Item"=w508)  [unwired: 1 out]
          n226 = xnode "FPGA I/O Node"("FPGA I/O In"=refnum<k21> "IO Socket\\SI 3 Deserializer GPIO 2 Input") -> ("I/O Item"=w507)  [unwired: 1 out]
          n227 = xnode "FPGA I/O Node"("FPGA I/O In"=refnum<k21> "IO Socket\\SI 3 Deserializer GPIO 3 Input") -> ("I/O Item"=w506)  [unwired: 1 out]
          n228 = xnode "FPGA I/O Node"("FPGA I/O In"=refnum<k21> "IO Socket\\SI 3 Deserializer GPIO 4 Input") -> ("I/O Item"=w505)  [unwired: 1 out]
          n229 = xnode "FPGA I/O Node"("FPGA I/O In"=refnum<k21> "IO Socket\\SI 3 Deserializer GPIO 5 Input") -> ("I/O Item"=w504)  [unwired: 1 out]
          n230 = xnode "FPGA I/O Node"("FPGA I/O In"=refnum<k21> "IO Socket\\SI 3 Deserializer GPIO 6 Input") -> ("I/O Item"=w502)  [unwired: 1 out]
          n231 = xnode "FPGA I/O Node"("FPGA I/O In"=refnum<k21> "IO Socket\\SI 3 Deserializer GPIO 7 Input") -> ("I/O Item"=w496)  [unwired: 1 out]
          n232 = xnode "FPGA I/O Node"("FPGA I/O In"=refnum<k21> "IO Socket\\SI 3 Deserializer GPIO 9 Input") -> ("I/O Item"=w497)  [unwired: 1 out]
          n233 = xnode "FPGA I/O Node"("FPGA I/O In"=refnum<k21> "IO Socket\\SI 3 Deserializer GPIO 10 Input") -> ("I/O Item"=w498)  [unwired: 1 out]
        }
        frame "SO 0 Serializer" {
          n234 = xnode "FPGA I/O Node"("FPGA I/O In"=refnum<k21> "IO Socket\\SO 0 Serializer GPIO 0 Input") -> ("I/O Item"=w519)  [unwired: 1 out]
          n235 = xnode "FPGA I/O Node"("FPGA I/O In"=refnum<k21> "IO Socket\\SO 0 Serializer GPIO 1 Input") -> ("I/O Item"=w518)  [unwired: 1 out]
          n236 = xnode "FPGA I/O Node"("FPGA I/O In"=refnum<k21> "IO Socket\\SO 0 Serializer GPIO 2 Input") -> ("I/O Item"=w517)  [unwired: 1 out]
          n237 = xnode "FPGA I/O Node"("FPGA I/O In"=refnum<k21> "IO Socket\\SO 0 Serializer GPIO 3 Input") -> ("I/O Item"=w516)  [unwired: 1 out]
        }
        frame "SO 1 Serializer" {
          n238 = xnode "FPGA I/O Node"("FPGA I/O In"=refnum<k21> "IO Socket\\SO 1 Serializer GPIO 0 Input") -> ("I/O Item"=w527)  [unwired: 1 out]
          n239 = xnode "FPGA I/O Node"("FPGA I/O In"=refnum<k21> "IO Socket\\SO 1 Serializer GPIO 1 Input") -> ("I/O Item"=w526)  [unwired: 1 out]
          n240 = xnode "FPGA I/O Node"("FPGA I/O In"=refnum<k21> "IO Socket\\SO 1 Serializer GPIO 2 Input") -> ("I/O Item"=w525)  [unwired: 1 out]
          n241 = xnode "FPGA I/O Node"("FPGA I/O In"=refnum<k21> "IO Socket\\SO 1 Serializer GPIO 3 Input") -> ("I/O Item"=w524)  [unwired: 1 out]
        }
        frame "SO 2 Serializer" {
          n242 = xnode "FPGA I/O Node"("FPGA I/O In"=refnum<k21> "IO Socket\\SO 2 Serializer GPIO 0 Input") -> ("I/O Item"=w535)  [unwired: 1 out]
          n243 = xnode "FPGA I/O Node"("FPGA I/O In"=refnum<k21> "IO Socket\\SO 2 Serializer GPIO 1 Input") -> ("I/O Item"=w534)  [unwired: 1 out]
          n244 = xnode "FPGA I/O Node"("FPGA I/O In"=refnum<k21> "IO Socket\\SO 2 Serializer GPIO 2 Input") -> ("I/O Item"=w533)  [unwired: 1 out]
          n245 = xnode "FPGA I/O Node"("FPGA I/O In"=refnum<k21> "IO Socket\\SO 2 Serializer GPIO 3 Input") -> ("I/O Item"=w532)  [unwired: 1 out]
        }
        frame "SO 3 Serializer" {
          n246 = xnode "FPGA I/O Node"("FPGA I/O In"=refnum<k21> "IO Socket\\SO 3 Serializer GPIO 0 Input") -> ("I/O Item"=w543)  [unwired: 1 out]
          n247 = xnode "FPGA I/O Node"("FPGA I/O In"=refnum<k21> "IO Socket\\SO 3 Serializer GPIO 1 Input") -> ("I/O Item"=w542)  [unwired: 1 out]
          n248 = xnode "FPGA I/O Node"("FPGA I/O In"=refnum<k21> "IO Socket\\SO 3 Serializer GPIO 2 Input") -> ("I/O Item"=w541)  [unwired: 1 out]
          n249 = xnode "FPGA I/O Node"("FPGA I/O In"=refnum<k21> "IO Socket\\SO 3 Serializer GPIO 3 Input") -> ("I/O Item"=w540)  [unwired: 1 out]
        }
      }
      n250 = Bundle By Name(cluster=T2 {"GPIO 0"=FALSE, "GPIO 1"=FALSE, "GPIO 2"=FALSE, "GPIO 3"=FALSE, "GPIO 4"=FALSE, "GPIO 5"=FALSE, "GPIO 6"=FALSE, "GPIO 7"=FALSE, "GPIO 8"=FALSE, "GPIO 9"=FALSE, "GPIO 10"=FALSE} ("gpio bank"), "GPIO 0"=w430, "GPIO 1"=w429, "GPIO 2"=w428, "GPIO 3"=w427, "GPIO 4"=w426, "GPIO 5"=w425, "GPIO 6"=w424, "GPIO 7"=w419, "GPIO 9"=w418, "GPIO 10"=w417) -> (w423:T2)
    }
    frame condition #6 {
      n251 = case shown="\"SI 0 SI 1 Deserializer\"" w555 {
        tunnel: [_ w583 w605 w627 w649] -> w550
        tunnel: [_ w582 w604 w626 w648] -> w562
        tunnel: [_ w581 w603 w625 w647] -> w561
        tunnel: [_ w580 w602 w624 w646] -> w560
        tunnel: [_ w579 w601 w623 w645] -> w559
        tunnel: [_ w578 w600 w622 w644] -> w558
        tunnel: [_ w576 w598 w620 w642] -> w557
        tunnel: [_ w572 w594 w616 w638] -> w554
        tunnel: [_ w571 w593 w615 w637] -> w553
        tunnel: [_ w570 w592 w614 w636] -> w552
        tunnel: [_ w569 w591 w613 w635] -> w551
        tunnel: w549 -> [w565 _ _ _ _]
        tunnel: [w564 _ _ _ _] -> w548
        frame Default {
          w564 = TRUE  # serdes id invalid
          n252 = case shown="True" w565 {
            frame False {
            }
            frame True {
              w567 = TRUE ("enable show error")
              # "Invalid GPIO bank select"
              n253 = call <instrlib>:"Assert.vi"("assert"=w567, "error code"=-1210, "enable show error"=w567) -> ()  [unwired: 13 in]
            }
          }
        }
        frame "SI 0 SI 1 Deserializer" {
          n254 = xnode "FPGA I/O Node"("FPGA I/O In"=refnum<k21> "IO Socket\\SI 0 SI 1 Deserializer MFP 0 Input") -> ("I/O Item"=w583)  [unwired: 1 out]
          n255 = xnode "FPGA I/O Node"("FPGA I/O In"=refnum<k21> "IO Socket\\SI 0 SI 1 Deserializer MFP 1 Input") -> ("I/O Item"=w582)  [unwired: 1 out]
          n256 = xnode "FPGA I/O Node"("FPGA I/O In"=refnum<k21> "IO Socket\\SI 0 SI 1 Deserializer MFP 2 Input") -> ("I/O Item"=w581)  [unwired: 1 out]
          n257 = xnode "FPGA I/O Node"("FPGA I/O In"=refnum<k21> "IO Socket\\SI 0 SI 1 Deserializer MFP 3 Input") -> ("I/O Item"=w580)  [unwired: 1 out]
          n258 = xnode "FPGA I/O Node"("FPGA I/O In"=refnum<k21> "IO Socket\\SI 0 SI 1 Deserializer MFP 4 Input") -> ("I/O Item"=w579)  [unwired: 1 out]
          n259 = xnode "FPGA I/O Node"("FPGA I/O In"=refnum<k21> "IO Socket\\SI 0 SI 1 Deserializer MFP 5 Input") -> ("I/O Item"=w578)  [unwired: 1 out]
          n260 = xnode "FPGA I/O Node"("FPGA I/O In"=refnum<k21> "IO Socket\\SI 0 SI 1 Deserializer MFP 6 Input") -> ("I/O Item"=w576)  [unwired: 1 out]
          n261 = xnode "FPGA I/O Node"("FPGA I/O In"=refnum<k21> "IO Socket\\SI 0 SI 1 Deserializer MFP 7 Input") -> ("I/O Item"=w572)  [unwired: 1 out]
          n262 = xnode "FPGA I/O Node"("FPGA I/O In"=refnum<k21> "IO Socket\\SI 0 SI 1 Deserializer MFP 8 Input") -> ("I/O Item"=w571)  [unwired: 1 out]
          n263 = xnode "FPGA I/O Node"("FPGA I/O In"=refnum<k21> "IO Socket\\SI 0 SI 1 Deserializer MFP 9 Input") -> ("I/O Item"=w570)  [unwired: 1 out]
          n264 = xnode "FPGA I/O Node"("FPGA I/O In"=refnum<k21> "IO Socket\\SI 0 SI 1 Deserializer MFP 10 Input") -> ("I/O Item"=w569)  [unwired: 1 out]
        }
        frame "SI 2 SI 3 Deserializer" {
          n265 = xnode "FPGA I/O Node"("FPGA I/O In"=refnum<k21> "IO Socket\\SI 2 SI 3 Deserializer MFP 0 Input") -> ("I/O Item"=w605)  [unwired: 1 out]
          n266 = xnode "FPGA I/O Node"("FPGA I/O In"=refnum<k21> "IO Socket\\SI 2 SI 3 Deserializer MFP 1 Input") -> ("I/O Item"=w604)  [unwired: 1 out]
          n267 = xnode "FPGA I/O Node"("FPGA I/O In"=refnum<k21> "IO Socket\\SI 2 SI 3 Deserializer MFP 2 Input") -> ("I/O Item"=w603)  [unwired: 1 out]
          n268 = xnode "FPGA I/O Node"("FPGA I/O In"=refnum<k21> "IO Socket\\SI 2 SI 3 Deserializer MFP 3 Input") -> ("I/O Item"=w602)  [unwired: 1 out]
          n269 = xnode "FPGA I/O Node"("FPGA I/O In"=refnum<k21> "IO Socket\\SI 2 SI 3 Deserializer MFP 4 Input") -> ("I/O Item"=w601)  [unwired: 1 out]
          n270 = xnode "FPGA I/O Node"("FPGA I/O In"=refnum<k21> "IO Socket\\SI 2 SI 3 Deserializer MFP 5 Input") -> ("I/O Item"=w600)  [unwired: 1 out]
          n271 = xnode "FPGA I/O Node"("FPGA I/O In"=refnum<k21> "IO Socket\\SI 2 SI 3 Deserializer MFP 6 Input") -> ("I/O Item"=w598)  [unwired: 1 out]
          n272 = xnode "FPGA I/O Node"("FPGA I/O In"=refnum<k21> "IO Socket\\SI 2 SI 3 Deserializer MFP 7 Input") -> ("I/O Item"=w594)  [unwired: 1 out]
          n273 = xnode "FPGA I/O Node"("FPGA I/O In"=refnum<k21> "IO Socket\\SI 2 SI 3 Deserializer MFP 8 Input") -> ("I/O Item"=w593)  [unwired: 1 out]
          n274 = xnode "FPGA I/O Node"("FPGA I/O In"=refnum<k21> "IO Socket\\SI 2 SI 3 Deserializer MFP 9 Input") -> ("I/O Item"=w592)  [unwired: 1 out]
          n275 = xnode "FPGA I/O Node"("FPGA I/O In"=refnum<k21> "IO Socket\\SI 2 SI 3 Deserializer MFP 10 Input") -> ("I/O Item"=w591)  [unwired: 1 out]
        }
        frame "SI 4 SI 5 Deserializer" {
          n276 = xnode "FPGA I/O Node"("FPGA I/O In"=refnum<k21> "IO Socket\\SI 4 SI 5 Deserializer MFP 0 Input") -> ("I/O Item"=w627)  [unwired: 1 out]
          n277 = xnode "FPGA I/O Node"("FPGA I/O In"=refnum<k21> "IO Socket\\SI 4 SI 5 Deserializer MFP 1 Input") -> ("I/O Item"=w626)  [unwired: 1 out]
          n278 = xnode "FPGA I/O Node"("FPGA I/O In"=refnum<k21> "IO Socket\\SI 4 SI 5 Deserializer MFP 2 Input") -> ("I/O Item"=w625)  [unwired: 1 out]
          n279 = xnode "FPGA I/O Node"("FPGA I/O In"=refnum<k21> "IO Socket\\SI 4 SI 5 Deserializer MFP 3 Input") -> ("I/O Item"=w624)  [unwired: 1 out]
          n280 = xnode "FPGA I/O Node"("FPGA I/O In"=refnum<k21> "IO Socket\\SI 4 SI 5 Deserializer MFP 4 Input") -> ("I/O Item"=w623)  [unwired: 1 out]
          n281 = xnode "FPGA I/O Node"("FPGA I/O In"=refnum<k21> "IO Socket\\SI 4 SI 5 Deserializer MFP 5 Input") -> ("I/O Item"=w622)  [unwired: 1 out]
          n282 = xnode "FPGA I/O Node"("FPGA I/O In"=refnum<k21> "IO Socket\\SI 4 SI 5 Deserializer MFP 6 Input") -> ("I/O Item"=w620)  [unwired: 1 out]
          n283 = xnode "FPGA I/O Node"("FPGA I/O In"=refnum<k21> "IO Socket\\SI 4 SI 5 Deserializer MFP 7 Input") -> ("I/O Item"=w616)  [unwired: 1 out]
          n284 = xnode "FPGA I/O Node"("FPGA I/O In"=refnum<k21> "IO Socket\\SI 4 SI 5 Deserializer MFP 8 Input") -> ("I/O Item"=w615)  [unwired: 1 out]
          n285 = xnode "FPGA I/O Node"("FPGA I/O In"=refnum<k21> "IO Socket\\SI 4 SI 5 Deserializer MFP 9 Input") -> ("I/O Item"=w614)  [unwired: 1 out]
          n286 = xnode "FPGA I/O Node"("FPGA I/O In"=refnum<k21> "IO Socket\\SI 4 SI 5 Deserializer MFP 10 Input") -> ("I/O Item"=w613)  [unwired: 1 out]
        }
        frame "SI 6 SI 7 Deserializer" {
          n287 = xnode "FPGA I/O Node"("FPGA I/O In"=refnum<k21> "IO Socket\\SI 6 SI 7 Deserializer MFP 0 Input") -> ("I/O Item"=w649)  [unwired: 1 out]
          n288 = xnode "FPGA I/O Node"("FPGA I/O In"=refnum<k21> "IO Socket\\SI 6 SI 7 Deserializer MFP 1 Input") -> ("I/O Item"=w648)  [unwired: 1 out]
          n289 = xnode "FPGA I/O Node"("FPGA I/O In"=refnum<k21> "IO Socket\\SI 6 SI 7 Deserializer MFP 2 Input") -> ("I/O Item"=w647)  [unwired: 1 out]
          n290 = xnode "FPGA I/O Node"("FPGA I/O In"=refnum<k21> "IO Socket\\SI 6 SI 7 Deserializer MFP 3 Input") -> ("I/O Item"=w646)  [unwired: 1 out]
          n291 = xnode "FPGA I/O Node"("FPGA I/O In"=refnum<k21> "IO Socket\\SI 6 SI 7 Deserializer MFP 4 Input") -> ("I/O Item"=w645)  [unwired: 1 out]
          n292 = xnode "FPGA I/O Node"("FPGA I/O In"=refnum<k21> "IO Socket\\SI 6 SI 7 Deserializer MFP 5 Input") -> ("I/O Item"=w644)  [unwired: 1 out]
          n293 = xnode "FPGA I/O Node"("FPGA I/O In"=refnum<k21> "IO Socket\\SI 6 SI 7 Deserializer MFP 6 Input") -> ("I/O Item"=w642)  [unwired: 1 out]
          n294 = xnode "FPGA I/O Node"("FPGA I/O In"=refnum<k21> "IO Socket\\SI 6 SI 7 Deserializer MFP 7 Input") -> ("I/O Item"=w638)  [unwired: 1 out]
          n295 = xnode "FPGA I/O Node"("FPGA I/O In"=refnum<k21> "IO Socket\\SI 6 SI 7 Deserializer MFP 8 Input") -> ("I/O Item"=w637)  [unwired: 1 out]
          n296 = xnode "FPGA I/O Node"("FPGA I/O In"=refnum<k21> "IO Socket\\SI 6 SI 7 Deserializer MFP 9 Input") -> ("I/O Item"=w636)  [unwired: 1 out]
          n297 = xnode "FPGA I/O Node"("FPGA I/O In"=refnum<k21> "IO Socket\\SI 6 SI 7 Deserializer MFP 10 Input") -> ("I/O Item"=w635)  [unwired: 1 out]
        }
      }
      n298 = Bundle By Name(cluster=T2 {"GPIO 0"=FALSE, "GPIO 1"=FALSE, "GPIO 2"=FALSE, "GPIO 3"=FALSE, "GPIO 4"=FALSE, "GPIO 5"=FALSE, "GPIO 6"=FALSE, "GPIO 7"=FALSE, "GPIO 8"=FALSE, "GPIO 9"=FALSE, "GPIO 10"=FALSE} ("gpio bank"), "GPIO 0"=w550, "GPIO 1"=w562, "GPIO 2"=w561, "GPIO 3"=w560, "GPIO 4"=w559, "GPIO 5"=w558, "GPIO 6"=w557, "GPIO 7"=w554, "GPIO 8"=w553, "GPIO 9"=w552, "GPIO 10"=w551) -> (w556:T2)
    }
    frame condition #7 {
      n299 = case shown="\"SI 0 SI 1 Deserializer\"" w663 {
        tunnel: [_ w691 w713] -> w658
        tunnel: [_ w690 w712] -> w670
        tunnel: [_ w689 w711] -> w669
        tunnel: [_ w688 w710] -> w668
        tunnel: [_ w687 w709] -> w667
        tunnel: [_ w686 w708] -> w666
        tunnel: [_ w684 w706] -> w665
        tunnel: [_ w680 w702] -> w662
        tunnel: [_ w679 w701] -> w661
        tunnel: [_ w678 w700] -> w660
        tunnel: [_ w677 w699] -> w659
        tunnel: w657 -> [w673 _ _]
        tunnel: [w672 _ _] -> w656
        frame Default {
          w672 = TRUE  # serdes id invalid
          n300 = case shown="True" w673 {
            frame False {
            }
            frame True {
              w675 = TRUE ("enable show error")
              # "Invalid GPIO bank select"
              n301 = call <instrlib>:"Assert.vi"("assert"=w675, "error code"=-1210, "enable show error"=w675) -> ()  [unwired: 13 in]
            }
          }
        }
        frame "SI 0 SI 1 Deserializer" {
          n302 = xnode "FPGA I/O Node"("FPGA I/O In"=refnum<k21> "IO Socket\\SI 0 SI 1 Deserializer MFP 0 Input") -> ("I/O Item"=w691)  [unwired: 1 out]
          n303 = xnode "FPGA I/O Node"("FPGA I/O In"=refnum<k21> "IO Socket\\SI 0 SI 1 Deserializer MFP 1 Input") -> ("I/O Item"=w690)  [unwired: 1 out]
          n304 = xnode "FPGA I/O Node"("FPGA I/O In"=refnum<k21> "IO Socket\\SI 0 SI 1 Deserializer MFP 2 Input") -> ("I/O Item"=w689)  [unwired: 1 out]
          n305 = xnode "FPGA I/O Node"("FPGA I/O In"=refnum<k21> "IO Socket\\SI 0 SI 1 Deserializer MFP 3 Input") -> ("I/O Item"=w688)  [unwired: 1 out]
          n306 = xnode "FPGA I/O Node"("FPGA I/O In"=refnum<k21> "IO Socket\\SI 0 SI 1 Deserializer MFP 4 Input") -> ("I/O Item"=w687)  [unwired: 1 out]
          n307 = xnode "FPGA I/O Node"("FPGA I/O In"=refnum<k21> "IO Socket\\SI 0 SI 1 Deserializer MFP 5 Input") -> ("I/O Item"=w686)  [unwired: 1 out]
          n308 = xnode "FPGA I/O Node"("FPGA I/O In"=refnum<k21> "IO Socket\\SI 0 SI 1 Deserializer MFP 6 Input") -> ("I/O Item"=w684)  [unwired: 1 out]
          n309 = xnode "FPGA I/O Node"("FPGA I/O In"=refnum<k21> "IO Socket\\SI 0 SI 1 Deserializer MFP 7 Input") -> ("I/O Item"=w680)  [unwired: 1 out]
          n310 = xnode "FPGA I/O Node"("FPGA I/O In"=refnum<k21> "IO Socket\\SI 0 SI 1 Deserializer MFP 8 Input") -> ("I/O Item"=w679)  [unwired: 1 out]
          n311 = xnode "FPGA I/O Node"("FPGA I/O In"=refnum<k21> "IO Socket\\SI 0 SI 1 Deserializer MFP 9 Input") -> ("I/O Item"=w678)  [unwired: 1 out]
          n312 = xnode "FPGA I/O Node"("FPGA I/O In"=refnum<k21> "IO Socket\\SI 0 SI 1 Deserializer MFP 10 Input") -> ("I/O Item"=w677)  [unwired: 1 out]
        }
        frame "SI 2 SI 3 Deserializer" {
          n313 = xnode "FPGA I/O Node"("FPGA I/O In"=refnum<k21> "IO Socket\\SI 2 SI 3 Deserializer MFP 0 Input") -> ("I/O Item"=w713)  [unwired: 1 out]
          n314 = xnode "FPGA I/O Node"("FPGA I/O In"=refnum<k21> "IO Socket\\SI 2 SI 3 Deserializer MFP 1 Input") -> ("I/O Item"=w712)  [unwired: 1 out]
          n315 = xnode "FPGA I/O Node"("FPGA I/O In"=refnum<k21> "IO Socket\\SI 2 SI 3 Deserializer MFP 2 Input") -> ("I/O Item"=w711)  [unwired: 1 out]
          n316 = xnode "FPGA I/O Node"("FPGA I/O In"=refnum<k21> "IO Socket\\SI 2 SI 3 Deserializer MFP 3 Input") -> ("I/O Item"=w710)  [unwired: 1 out]
          n317 = xnode "FPGA I/O Node"("FPGA I/O In"=refnum<k21> "IO Socket\\SI 2 SI 3 Deserializer MFP 4 Input") -> ("I/O Item"=w709)  [unwired: 1 out]
          n318 = xnode "FPGA I/O Node"("FPGA I/O In"=refnum<k21> "IO Socket\\SI 2 SI 3 Deserializer MFP 5 Input") -> ("I/O Item"=w708)  [unwired: 1 out]
          n319 = xnode "FPGA I/O Node"("FPGA I/O In"=refnum<k21> "IO Socket\\SI 2 SI 3 Deserializer MFP 6 Input") -> ("I/O Item"=w706)  [unwired: 1 out]
          n320 = xnode "FPGA I/O Node"("FPGA I/O In"=refnum<k21> "IO Socket\\SI 2 SI 3 Deserializer MFP 7 Input") -> ("I/O Item"=w702)  [unwired: 1 out]
          n321 = xnode "FPGA I/O Node"("FPGA I/O In"=refnum<k21> "IO Socket\\SI 2 SI 3 Deserializer MFP 8 Input") -> ("I/O Item"=w701)  [unwired: 1 out]
          n322 = xnode "FPGA I/O Node"("FPGA I/O In"=refnum<k21> "IO Socket\\SI 2 SI 3 Deserializer MFP 9 Input") -> ("I/O Item"=w700)  [unwired: 1 out]
          n323 = xnode "FPGA I/O Node"("FPGA I/O In"=refnum<k21> "IO Socket\\SI 2 SI 3 Deserializer MFP 10 Input") -> ("I/O Item"=w699)  [unwired: 1 out]
        }
      }
      n324 = Bundle By Name(cluster=T2 {"GPIO 0"=FALSE, "GPIO 1"=FALSE, "GPIO 2"=FALSE, "GPIO 3"=FALSE, "GPIO 4"=FALSE, "GPIO 5"=FALSE, "GPIO 6"=FALSE, "GPIO 7"=FALSE, "GPIO 8"=FALSE, "GPIO 9"=FALSE, "GPIO 10"=FALSE} ("gpio bank"), "GPIO 0"=w658, "GPIO 1"=w670, "GPIO 2"=w669, "GPIO 3"=w668, "GPIO 4"=w667, "GPIO 5"=w666, "GPIO 6"=w665, "GPIO 7"=w662, "GPIO 8"=w661, "GPIO 9"=w660, "GPIO 10"=w659) -> (w664:T2)
    }
    frame condition #8 {
      n325 = case shown="Default" w724 {
        tunnel: [_ w748 w764 w780 w796 w812 w828 w844 w860] -> w731
        tunnel: [_ w747 w763 w779 w795 w811 w827 w843 w859] -> w730
        tunnel: [_ w746 w762 w778 w794 w810 w826 w842 w858] -> w729
        tunnel: [_ w745 w761 w777 w793 w809 w825 w841 w857] -> w728
        tunnel: [_ w741 w757 w773 w789 w805 w821 w837 w853] -> w727
        tunnel: [_ w740 w756 w772 w788 w804 w820 w836 w852] -> w726
        tunnel: [_ w739 w755 w771 w787 w803 w819 w835 w851] -> w723
        tunnel: [_ w737 w753 w769 w785 w801 w817 w833 w849] -> w722
        tunnel: w721 -> [w734 _ _ _ _ _ _ _ _]
        tunnel: [w733 _ _ _ _ _ _ _ _] -> w720
        frame Default {
          w733 = TRUE  # serdes id invalid
          n326 = case shown="True" w734 {
            frame False {
            }
            frame True {
              w736 = TRUE ("enable show error")
              # "Invalid GPIO bank select"
              n327 = call <instrlib>:"Assert.vi"("assert"=w736, "error code"=-1210, "enable show error"=w736) -> ()  [unwired: 13 in]
            }
          }
        }
        frame "SO 0 Serializer" {
          n328 = xnode "FPGA I/O Node"("FPGA I/O In"=refnum<k21> "IO Socket\\SO 0 Serializer MFP 0 Input") -> ("I/O Item"=w748)  [unwired: 1 out]
          n329 = xnode "FPGA I/O Node"("FPGA I/O In"=refnum<k21> "IO Socket\\SO 0 Serializer MFP 1 Input") -> ("I/O Item"=w747)  [unwired: 1 out]
          n330 = xnode "FPGA I/O Node"("FPGA I/O In"=refnum<k21> "IO Socket\\SO 0 Serializer MFP 2 Input") -> ("I/O Item"=w746)  [unwired: 1 out]
          n331 = xnode "FPGA I/O Node"("FPGA I/O In"=refnum<k21> "IO Socket\\SO 0 Serializer MFP 3 Input") -> ("I/O Item"=w745)  [unwired: 1 out]
          n332 = xnode "FPGA I/O Node"("FPGA I/O In"=refnum<k21> "IO Socket\\SO 0 Serializer MFP 4 Input") -> ("I/O Item"=w741)  [unwired: 1 out]
          n333 = xnode "FPGA I/O Node"("FPGA I/O In"=refnum<k21> "IO Socket\\SO 0 Serializer MFP 6 Input") -> ("I/O Item"=w740)  [unwired: 1 out]
          n334 = xnode "FPGA I/O Node"("FPGA I/O In"=refnum<k21> "IO Socket\\SO 0 Serializer MFP 7 Input") -> ("I/O Item"=w739)  [unwired: 1 out]
          n335 = xnode "FPGA I/O Node"("FPGA I/O In"=refnum<k21> "IO Socket\\SO 0 Serializer MFP 8 Input") -> ("I/O Item"=w737)  [unwired: 1 out]
        }
        frame "SO 1 Serializer" {
          n336 = xnode "FPGA I/O Node"("FPGA I/O In"=refnum<k21> "IO Socket\\SO 1 Serializer MFP 0 Input") -> ("I/O Item"=w764)  [unwired: 1 out]
          n337 = xnode "FPGA I/O Node"("FPGA I/O In"=refnum<k21> "IO Socket\\SO 1 Serializer MFP 1 Input") -> ("I/O Item"=w763)  [unwired: 1 out]
          n338 = xnode "FPGA I/O Node"("FPGA I/O In"=refnum<k21> "IO Socket\\SO 1 Serializer MFP 2 Input") -> ("I/O Item"=w762)  [unwired: 1 out]
          n339 = xnode "FPGA I/O Node"("FPGA I/O In"=refnum<k21> "IO Socket\\SO 1 Serializer MFP 3 Input") -> ("I/O Item"=w761)  [unwired: 1 out]
          n340 = xnode "FPGA I/O Node"("FPGA I/O In"=refnum<k21> "IO Socket\\SO 1 Serializer MFP 4 Input") -> ("I/O Item"=w757)  [unwired: 1 out]
          n341 = xnode "FPGA I/O Node"("FPGA I/O In"=refnum<k21> "IO Socket\\SO 1 Serializer MFP 6 Input") -> ("I/O Item"=w756)  [unwired: 1 out]
          n342 = xnode "FPGA I/O Node"("FPGA I/O In"=refnum<k21> "IO Socket\\SO 1 Serializer MFP 7 Input") -> ("I/O Item"=w755)  [unwired: 1 out]
          n343 = xnode "FPGA I/O Node"("FPGA I/O In"=refnum<k21> "IO Socket\\SO 1 Serializer MFP 8 Input") -> ("I/O Item"=w753)  [unwired: 1 out]
        }
        frame "SO 2 Serializer" {
          n344 = xnode "FPGA I/O Node"("FPGA I/O In"=refnum<k21> "IO Socket\\SO 2 Serializer MFP 0 Input") -> ("I/O Item"=w780)  [unwired: 1 out]
          n345 = xnode "FPGA I/O Node"("FPGA I/O In"=refnum<k21> "IO Socket\\SO 2 Serializer MFP 1 Input") -> ("I/O Item"=w779)  [unwired: 1 out]
          n346 = xnode "FPGA I/O Node"("FPGA I/O In"=refnum<k21> "IO Socket\\SO 2 Serializer MFP 2 Input") -> ("I/O Item"=w778)  [unwired: 1 out]
          n347 = xnode "FPGA I/O Node"("FPGA I/O In"=refnum<k21> "IO Socket\\SO 2 Serializer MFP 3 Input") -> ("I/O Item"=w777)  [unwired: 1 out]
          n348 = xnode "FPGA I/O Node"("FPGA I/O In"=refnum<k21> "IO Socket\\SO 2 Serializer MFP 4 Input") -> ("I/O Item"=w773)  [unwired: 1 out]
          n349 = xnode "FPGA I/O Node"("FPGA I/O In"=refnum<k21> "IO Socket\\SO 2 Serializer MFP 6 Input") -> ("I/O Item"=w772)  [unwired: 1 out]
          n350 = xnode "FPGA I/O Node"("FPGA I/O In"=refnum<k21> "IO Socket\\SO 2 Serializer MFP 7 Input") -> ("I/O Item"=w771)  [unwired: 1 out]
          n351 = xnode "FPGA I/O Node"("FPGA I/O In"=refnum<k21> "IO Socket\\SO 2 Serializer MFP 8 Input") -> ("I/O Item"=w769)  [unwired: 1 out]
        }
        frame "SO 3 Serializer" {
          n352 = xnode "FPGA I/O Node"("FPGA I/O In"=refnum<k21> "IO Socket\\SO 3 Serializer MFP 0 Input") -> ("I/O Item"=w796)  [unwired: 1 out]
          n353 = xnode "FPGA I/O Node"("FPGA I/O In"=refnum<k21> "IO Socket\\SO 3 Serializer MFP 1 Input") -> ("I/O Item"=w795)  [unwired: 1 out]
          n354 = xnode "FPGA I/O Node"("FPGA I/O In"=refnum<k21> "IO Socket\\SO 3 Serializer MFP 2 Input") -> ("I/O Item"=w794)  [unwired: 1 out]
          n355 = xnode "FPGA I/O Node"("FPGA I/O In"=refnum<k21> "IO Socket\\SO 3 Serializer MFP 3 Input") -> ("I/O Item"=w793)  [unwired: 1 out]
          n356 = xnode "FPGA I/O Node"("FPGA I/O In"=refnum<k21> "IO Socket\\SO 3 Serializer MFP 4 Input") -> ("I/O Item"=w789)  [unwired: 1 out]
          n357 = xnode "FPGA I/O Node"("FPGA I/O In"=refnum<k21> "IO Socket\\SO 3 Serializer MFP 6 Input") -> ("I/O Item"=w788)  [unwired: 1 out]
          n358 = xnode "FPGA I/O Node"("FPGA I/O In"=refnum<k21> "IO Socket\\SO 3 Serializer MFP 7 Input") -> ("I/O Item"=w787)  [unwired: 1 out]
          n359 = xnode "FPGA I/O Node"("FPGA I/O In"=refnum<k21> "IO Socket\\SO 3 Serializer MFP 8 Input") -> ("I/O Item"=w785)  [unwired: 1 out]
        }
        frame "SO 4 Serializer" {
          n360 = xnode "FPGA I/O Node"("FPGA I/O In"=refnum<k21> "IO Socket\\SO 4 Serializer MFP 0 Input") -> ("I/O Item"=w812)  [unwired: 1 out]
          n361 = xnode "FPGA I/O Node"("FPGA I/O In"=refnum<k21> "IO Socket\\SO 4 Serializer MFP 1 Input") -> ("I/O Item"=w811)  [unwired: 1 out]
          n362 = xnode "FPGA I/O Node"("FPGA I/O In"=refnum<k21> "IO Socket\\SO 4 Serializer MFP 2 Input") -> ("I/O Item"=w810)  [unwired: 1 out]
          n363 = xnode "FPGA I/O Node"("FPGA I/O In"=refnum<k21> "IO Socket\\SO 4 Serializer MFP 3 Input") -> ("I/O Item"=w809)  [unwired: 1 out]
          n364 = xnode "FPGA I/O Node"("FPGA I/O In"=refnum<k21> "IO Socket\\SO 4 Serializer MFP 4 Input") -> ("I/O Item"=w805)  [unwired: 1 out]
          n365 = xnode "FPGA I/O Node"("FPGA I/O In"=refnum<k21> "IO Socket\\SO 4 Serializer MFP 6 Input") -> ("I/O Item"=w804)  [unwired: 1 out]
          n366 = xnode "FPGA I/O Node"("FPGA I/O In"=refnum<k21> "IO Socket\\SO 4 Serializer MFP 7 Input") -> ("I/O Item"=w803)  [unwired: 1 out]
          n367 = xnode "FPGA I/O Node"("FPGA I/O In"=refnum<k21> "IO Socket\\SO 4 Serializer MFP 8 Input") -> ("I/O Item"=w801)  [unwired: 1 out]
        }
        frame "SO 5 Serializer" {
          n368 = xnode "FPGA I/O Node"("FPGA I/O In"=refnum<k21> "IO Socket\\SO 5 Serializer MFP 0 Input") -> ("I/O Item"=w828)  [unwired: 1 out]
          n369 = xnode "FPGA I/O Node"("FPGA I/O In"=refnum<k21> "IO Socket\\SO 5 Serializer MFP 1 Input") -> ("I/O Item"=w827)  [unwired: 1 out]
          n370 = xnode "FPGA I/O Node"("FPGA I/O In"=refnum<k21> "IO Socket\\SO 5 Serializer MFP 2 Input") -> ("I/O Item"=w826)  [unwired: 1 out]
          n371 = xnode "FPGA I/O Node"("FPGA I/O In"=refnum<k21> "IO Socket\\SO 5 Serializer MFP 3 Input") -> ("I/O Item"=w825)  [unwired: 1 out]
          n372 = xnode "FPGA I/O Node"("FPGA I/O In"=refnum<k21> "IO Socket\\SO 5 Serializer MFP 4 Input") -> ("I/O Item"=w821)  [unwired: 1 out]
          n373 = xnode "FPGA I/O Node"("FPGA I/O In"=refnum<k21> "IO Socket\\SO 5 Serializer MFP 6 Input") -> ("I/O Item"=w820)  [unwired: 1 out]
          n374 = xnode "FPGA I/O Node"("FPGA I/O In"=refnum<k21> "IO Socket\\SO 5 Serializer MFP 7 Input") -> ("I/O Item"=w819)  [unwired: 1 out]
          n375 = xnode "FPGA I/O Node"("FPGA I/O In"=refnum<k21> "IO Socket\\SO 5 Serializer MFP 8 Input") -> ("I/O Item"=w817)  [unwired: 1 out]
        }
        frame "SO 6 Serializer" {
          n376 = xnode "FPGA I/O Node"("FPGA I/O In"=refnum<k21> "IO Socket\\SO 6 Serializer MFP 0 Input") -> ("I/O Item"=w844)  [unwired: 1 out]
          n377 = xnode "FPGA I/O Node"("FPGA I/O In"=refnum<k21> "IO Socket\\SO 6 Serializer MFP 1 Input") -> ("I/O Item"=w843)  [unwired: 1 out]
          n378 = xnode "FPGA I/O Node"("FPGA I/O In"=refnum<k21> "IO Socket\\SO 6 Serializer MFP 2 Input") -> ("I/O Item"=w842)  [unwired: 1 out]
          n379 = xnode "FPGA I/O Node"("FPGA I/O In"=refnum<k21> "IO Socket\\SO 6 Serializer MFP 3 Input") -> ("I/O Item"=w841)  [unwired: 1 out]
          n380 = xnode "FPGA I/O Node"("FPGA I/O In"=refnum<k21> "IO Socket\\SO 6 Serializer MFP 4 Input") -> ("I/O Item"=w837)  [unwired: 1 out]
          n381 = xnode "FPGA I/O Node"("FPGA I/O In"=refnum<k21> "IO Socket\\SO 6 Serializer MFP 6 Input") -> ("I/O Item"=w836)  [unwired: 1 out]
          n382 = xnode "FPGA I/O Node"("FPGA I/O In"=refnum<k21> "IO Socket\\SO 6 Serializer MFP 7 Input") -> ("I/O Item"=w835)  [unwired: 1 out]
          n383 = xnode "FPGA I/O Node"("FPGA I/O In"=refnum<k21> "IO Socket\\SO 6 Serializer MFP 8 Input") -> ("I/O Item"=w833)  [unwired: 1 out]
        }
        frame "SO 7 Serializer" {
          n384 = xnode "FPGA I/O Node"("FPGA I/O In"=refnum<k21> "IO Socket\\SO 7 Serializer MFP 0 Input") -> ("I/O Item"=w860)  [unwired: 1 out]
          n385 = xnode "FPGA I/O Node"("FPGA I/O In"=refnum<k21> "IO Socket\\SO 7 Serializer MFP 1 Input") -> ("I/O Item"=w859)  [unwired: 1 out]
          n386 = xnode "FPGA I/O Node"("FPGA I/O In"=refnum<k21> "IO Socket\\SO 7 Serializer MFP 2 Input") -> ("I/O Item"=w858)  [unwired: 1 out]
          n387 = xnode "FPGA I/O Node"("FPGA I/O In"=refnum<k21> "IO Socket\\SO 7 Serializer MFP 3 Input") -> ("I/O Item"=w857)  [unwired: 1 out]
          n388 = xnode "FPGA I/O Node"("FPGA I/O In"=refnum<k21> "IO Socket\\SO 7 Serializer MFP 4 Input") -> ("I/O Item"=w853)  [unwired: 1 out]
          n389 = xnode "FPGA I/O Node"("FPGA I/O In"=refnum<k21> "IO Socket\\SO 7 Serializer MFP 6 Input") -> ("I/O Item"=w852)  [unwired: 1 out]
          n390 = xnode "FPGA I/O Node"("FPGA I/O In"=refnum<k21> "IO Socket\\SO 7 Serializer MFP 7 Input") -> ("I/O Item"=w851)  [unwired: 1 out]
          n391 = xnode "FPGA I/O Node"("FPGA I/O In"=refnum<k21> "IO Socket\\SO 7 Serializer MFP 8 Input") -> ("I/O Item"=w849)  [unwired: 1 out]
        }
      }
      n392 = Bundle By Name(cluster=T2 {"GPIO 0"=FALSE, "GPIO 1"=FALSE, "GPIO 2"=FALSE, "GPIO 3"=FALSE, "GPIO 4"=FALSE, "GPIO 5"=FALSE, "GPIO 6"=FALSE, "GPIO 7"=FALSE, "GPIO 8"=FALSE, "GPIO 9"=FALSE, "GPIO 10"=FALSE} ("gpio bank"), "GPIO 0"=w731, "GPIO 1"=w730, "GPIO 2"=w729, "GPIO 3"=w728, "GPIO 4"=w727, "GPIO 6"=w726, "GPIO 7"=w723, "GPIO 8"=w722) -> (w725:T2)
    }
    frame condition #9 {
      n393 = case shown="\"SO 1 Serializer\"" w869 {
        tunnel: [_ w893 w909 w925 w941] -> w876
        tunnel: [_ w892 w908 w924 w940] -> w875
        tunnel: [_ w891 w907 w923 w939] -> w874
        tunnel: [_ w890 w906 w922 w938] -> w873
        tunnel: [_ w886 w902 w918 w934] -> w872
        tunnel: [_ w885 w901 w917 w933] -> w871
        tunnel: [_ w884 w900 w916 w932] -> w868
        tunnel: [_ w882 w898 w914 w930] -> w867
        tunnel: w866 -> [w879 _ _ _ _]
        tunnel: [w878 _ _ _ _] -> w865
        frame Default {
          w878 = TRUE  # serdes id invalid
          n394 = case shown="True" w879 {
            frame False {
            }
            frame True {
              w881 = TRUE ("enable show error")
              # "Invalid GPIO bank select"
              n395 = call <instrlib>:"Assert.vi"("assert"=w881, "error code"=-1210, "enable show error"=w881) -> ()  [unwired: 13 in]
            }
          }
        }
        frame "SO 0 Serializer" {
          n396 = xnode "FPGA I/O Node"("FPGA I/O In"=refnum<k21> "IO Socket\\SO 0 Serializer MFP 0 Input") -> ("I/O Item"=w893)  [unwired: 1 out]
          n397 = xnode "FPGA I/O Node"("FPGA I/O In"=refnum<k21> "IO Socket\\SO 0 Serializer MFP 1 Input") -> ("I/O Item"=w892)  [unwired: 1 out]
          n398 = xnode "FPGA I/O Node"("FPGA I/O In"=refnum<k21> "IO Socket\\SO 0 Serializer MFP 2 Input") -> ("I/O Item"=w891)  [unwired: 1 out]
          n399 = xnode "FPGA I/O Node"("FPGA I/O In"=refnum<k21> "IO Socket\\SO 0 Serializer MFP 3 Input") -> ("I/O Item"=w890)  [unwired: 1 out]
          n400 = xnode "FPGA I/O Node"("FPGA I/O In"=refnum<k21> "IO Socket\\SO 0 Serializer MFP 4 Input") -> ("I/O Item"=w886)  [unwired: 1 out]
          n401 = xnode "FPGA I/O Node"("FPGA I/O In"=refnum<k21> "IO Socket\\SO 0 Serializer MFP 6 Input") -> ("I/O Item"=w885)  [unwired: 1 out]
          n402 = xnode "FPGA I/O Node"("FPGA I/O In"=refnum<k21> "IO Socket\\SO 0 Serializer MFP 7 Input") -> ("I/O Item"=w884)  [unwired: 1 out]
          n403 = xnode "FPGA I/O Node"("FPGA I/O In"=refnum<k21> "IO Socket\\SO 0 Serializer MFP 8 Input") -> ("I/O Item"=w882)  [unwired: 1 out]
        }
        frame "SO 1 Serializer" {
          n404 = xnode "FPGA I/O Node"("FPGA I/O In"=refnum<k21> "IO Socket\\SO 1 Serializer MFP 0 Input") -> ("I/O Item"=w909)  [unwired: 1 out]
          n405 = xnode "FPGA I/O Node"("FPGA I/O In"=refnum<k21> "IO Socket\\SO 1 Serializer MFP 1 Input") -> ("I/O Item"=w908)  [unwired: 1 out]
          n406 = xnode "FPGA I/O Node"("FPGA I/O In"=refnum<k21> "IO Socket\\SO 1 Serializer MFP 2 Input") -> ("I/O Item"=w907)  [unwired: 1 out]
          n407 = xnode "FPGA I/O Node"("FPGA I/O In"=refnum<k21> "IO Socket\\SO 1 Serializer MFP 3 Input") -> ("I/O Item"=w906)  [unwired: 1 out]
          n408 = xnode "FPGA I/O Node"("FPGA I/O In"=refnum<k21> "IO Socket\\SO 1 Serializer MFP 4 Input") -> ("I/O Item"=w902)  [unwired: 1 out]
          n409 = xnode "FPGA I/O Node"("FPGA I/O In"=refnum<k21> "IO Socket\\SO 1 Serializer MFP 6 Input") -> ("I/O Item"=w901)  [unwired: 1 out]
          n410 = xnode "FPGA I/O Node"("FPGA I/O In"=refnum<k21> "IO Socket\\SO 1 Serializer MFP 7 Input") -> ("I/O Item"=w900)  [unwired: 1 out]
          n411 = xnode "FPGA I/O Node"("FPGA I/O In"=refnum<k21> "IO Socket\\SO 1 Serializer MFP 8 Input") -> ("I/O Item"=w898)  [unwired: 1 out]
        }
        frame "SO 2 Serializer" {
          n412 = xnode "FPGA I/O Node"("FPGA I/O In"=refnum<k21> "IO Socket\\SO 2 Serializer MFP 0 Input") -> ("I/O Item"=w925)  [unwired: 1 out]
          n413 = xnode "FPGA I/O Node"("FPGA I/O In"=refnum<k21> "IO Socket\\SO 2 Serializer MFP 1 Input") -> ("I/O Item"=w924)  [unwired: 1 out]
          n414 = xnode "FPGA I/O Node"("FPGA I/O In"=refnum<k21> "IO Socket\\SO 2 Serializer MFP 2 Input") -> ("I/O Item"=w923)  [unwired: 1 out]
          n415 = xnode "FPGA I/O Node"("FPGA I/O In"=refnum<k21> "IO Socket\\SO 2 Serializer MFP 3 Input") -> ("I/O Item"=w922)  [unwired: 1 out]
          n416 = xnode "FPGA I/O Node"("FPGA I/O In"=refnum<k21> "IO Socket\\SO 2 Serializer MFP 4 Input") -> ("I/O Item"=w918)  [unwired: 1 out]
          n417 = xnode "FPGA I/O Node"("FPGA I/O In"=refnum<k21> "IO Socket\\SO 2 Serializer MFP 6 Input") -> ("I/O Item"=w917)  [unwired: 1 out]
          n418 = xnode "FPGA I/O Node"("FPGA I/O In"=refnum<k21> "IO Socket\\SO 2 Serializer MFP 7 Input") -> ("I/O Item"=w916)  [unwired: 1 out]
          n419 = xnode "FPGA I/O Node"("FPGA I/O In"=refnum<k21> "IO Socket\\SO 2 Serializer MFP 8 Input") -> ("I/O Item"=w914)  [unwired: 1 out]
        }
        frame "SO 3 Serializer" {
          n420 = xnode "FPGA I/O Node"("FPGA I/O In"=refnum<k21> "IO Socket\\SO 3 Serializer MFP 0 Input") -> ("I/O Item"=w941)  [unwired: 1 out]
          n421 = xnode "FPGA I/O Node"("FPGA I/O In"=refnum<k21> "IO Socket\\SO 3 Serializer MFP 1 Input") -> ("I/O Item"=w940)  [unwired: 1 out]
          n422 = xnode "FPGA I/O Node"("FPGA I/O In"=refnum<k21> "IO Socket\\SO 3 Serializer MFP 2 Input") -> ("I/O Item"=w939)  [unwired: 1 out]
          n423 = xnode "FPGA I/O Node"("FPGA I/O In"=refnum<k21> "IO Socket\\SO 3 Serializer MFP 3 Input") -> ("I/O Item"=w938)  [unwired: 1 out]
          n424 = xnode "FPGA I/O Node"("FPGA I/O In"=refnum<k21> "IO Socket\\SO 3 Serializer MFP 4 Input") -> ("I/O Item"=w934)  [unwired: 1 out]
          n425 = xnode "FPGA I/O Node"("FPGA I/O In"=refnum<k21> "IO Socket\\SO 3 Serializer MFP 6 Input") -> ("I/O Item"=w933)  [unwired: 1 out]
          n426 = xnode "FPGA I/O Node"("FPGA I/O In"=refnum<k21> "IO Socket\\SO 3 Serializer MFP 7 Input") -> ("I/O Item"=w932)  [unwired: 1 out]
          n427 = xnode "FPGA I/O Node"("FPGA I/O In"=refnum<k21> "IO Socket\\SO 3 Serializer MFP 8 Input") -> ("I/O Item"=w930)  [unwired: 1 out]
        }
      }
      n428 = Bundle By Name(cluster=T2 {"GPIO 0"=FALSE, "GPIO 1"=FALSE, "GPIO 2"=FALSE, "GPIO 3"=FALSE, "GPIO 4"=FALSE, "GPIO 5"=FALSE, "GPIO 6"=FALSE, "GPIO 7"=FALSE, "GPIO 8"=FALSE, "GPIO 9"=FALSE, "GPIO 10"=FALSE} ("gpio bank"), "GPIO 0"=w876, "GPIO 1"=w875, "GPIO 2"=w874, "GPIO 3"=w873, "GPIO 4"=w872, "GPIO 6"=w871, "GPIO 7"=w868, "GPIO 8"=w867) -> (w870:T2)
    }
    frame condition #10 {
      n429 = case shown="\"SI 0 Deserializer\"" w952 {
        tunnel: [_ w981 w1003 w1025 w1047 w1065 w1081 w1097 w1113] -> w960
        tunnel: [_ w980 w1002 w1024 w1046 w1064 w1080 w1096 w1112] -> w959
        tunnel: [_ w979 w1001 w1023 w1045 w1063 w1079 w1095 w1111] -> w958
        tunnel: [_ w978 w1000 w1022 w1044 w1062 w1078 w1094 w1110] -> w957
        tunnel: [_ w977 w999 w1021 w1043 w1058 w1074 w1090 w1106] -> w956
        tunnel: [_ w976 w998 w1020 w1042 _ _ _ _] -> w955
        tunnel: [_ w974 w996 w1018 w1040 w1057 w1073 w1089 w1105] -> w954
        tunnel: [_ w972 w994 w1016 w1038 w1056 w1072 w1088 w1104] -> w951
        tunnel: [_ w969 w991 w1013 w1032 w1054 w1070 w1086 w1102] -> w950
        tunnel: w949 -> [w963 _ _ _ _ _ _ _ _]
        tunnel: [w962 _ _ _ _ _ _ _ _] -> w948
        tunnel: [_ w967 w988 w1011 w1035 _ _ _ _] -> w947
        tunnel: [_ w966 w989 w1010 w1034 _ _ _ _] -> w946
        frame Default {
          w962 = TRUE  # serdes id invalid
          n430 = case shown="True" w963 {
            frame False {
            }
            frame True {
              w965 = TRUE ("enable show error")
              # "Invalid GPIO bank select"
              n431 = call <instrlib>:"Assert.vi"("assert"=w965, "error code"=-1210, "enable show error"=w965) -> ()  [unwired: 13 in]
            }
          }
        }
        frame "SI 0 Deserializer" {
          n432 = xnode "FPGA I/O Node"("FPGA I/O In"=refnum<k21> "IO Socket\\SI 0 Deserializer MFP 0 Input") -> ("I/O Item"=w981)  [unwired: 1 out]
          n433 = xnode "FPGA I/O Node"("FPGA I/O In"=refnum<k21> "IO Socket\\SI 0 Deserializer MFP 1 Input") -> ("I/O Item"=w980)  [unwired: 1 out]
          n434 = xnode "FPGA I/O Node"("FPGA I/O In"=refnum<k21> "IO Socket\\SI 0 Deserializer MFP 2 Input") -> ("I/O Item"=w979)  [unwired: 1 out]
          n435 = xnode "FPGA I/O Node"("FPGA I/O In"=refnum<k21> "IO Socket\\SI 0 Deserializer MFP 3 Input") -> ("I/O Item"=w978)  [unwired: 1 out]
          n436 = xnode "FPGA I/O Node"("FPGA I/O In"=refnum<k21> "IO Socket\\SI 0 Deserializer MFP 4 Input") -> ("I/O Item"=w977)  [unwired: 1 out]
          n437 = xnode "FPGA I/O Node"("FPGA I/O In"=refnum<k21> "IO Socket\\SI 0 Deserializer MFP 5 Input") -> ("I/O Item"=w976)  [unwired: 1 out]
          n438 = xnode "FPGA I/O Node"("FPGA I/O In"=refnum<k21> "IO Socket\\SI 0 Deserializer MFP 6 Input") -> ("I/O Item"=w974)  [unwired: 1 out]
          n439 = xnode "FPGA I/O Node"("FPGA I/O In"=refnum<k21> "IO Socket\\SI 0 Deserializer MFP 7 Input") -> ("I/O Item"=w972)  [unwired: 1 out]
          n440 = xnode "FPGA I/O Node"("FPGA I/O In"=refnum<k21> "IO Socket\\SI 0 Deserializer MFP 8 Input") -> ("I/O Item"=w969)  [unwired: 1 out]
          n441 = xnode "FPGA I/O Node"("FPGA I/O In"=refnum<k21> "IO Socket\\SI 0 Deserializer MFP 9 Input") -> ("I/O Item"=w967)  [unwired: 1 out]
          n442 = xnode "FPGA I/O Node"("FPGA I/O In"=refnum<k21> "IO Socket\\SI 0 Deserializer MFP 10 Input") -> ("I/O Item"=w966)  [unwired: 1 out]
        }
        frame "SI 1 Deserializer" {
          n443 = xnode "FPGA I/O Node"("FPGA I/O In"=refnum<k21> "IO Socket\\SI 1 Deserializer MFP 0 Input") -> ("I/O Item"=w1003)  [unwired: 1 out]
          n444 = xnode "FPGA I/O Node"("FPGA I/O In"=refnum<k21> "IO Socket\\SI 1 Deserializer MFP 1 Input") -> ("I/O Item"=w1002)  [unwired: 1 out]
          n445 = xnode "FPGA I/O Node"("FPGA I/O In"=refnum<k21> "IO Socket\\SI 1 Deserializer MFP 2 Input") -> ("I/O Item"=w1001)  [unwired: 1 out]
          n446 = xnode "FPGA I/O Node"("FPGA I/O In"=refnum<k21> "IO Socket\\SI 1 Deserializer MFP 3 Input") -> ("I/O Item"=w1000)  [unwired: 1 out]
          n447 = xnode "FPGA I/O Node"("FPGA I/O In"=refnum<k21> "IO Socket\\SI 1 Deserializer MFP 4 Input") -> ("I/O Item"=w999)  [unwired: 1 out]
          n448 = xnode "FPGA I/O Node"("FPGA I/O In"=refnum<k21> "IO Socket\\SI 1 Deserializer MFP 5 Input") -> ("I/O Item"=w998)  [unwired: 1 out]
          n449 = xnode "FPGA I/O Node"("FPGA I/O In"=refnum<k21> "IO Socket\\SI 1 Deserializer MFP 6 Input") -> ("I/O Item"=w996)  [unwired: 1 out]
          n450 = xnode "FPGA I/O Node"("FPGA I/O In"=refnum<k21> "IO Socket\\SI 1 Deserializer MFP 7 Input") -> ("I/O Item"=w994)  [unwired: 1 out]
          n451 = xnode "FPGA I/O Node"("FPGA I/O In"=refnum<k21> "IO Socket\\SI 1 Deserializer MFP 8 Input") -> ("I/O Item"=w991)  [unwired: 1 out]
          n452 = xnode "FPGA I/O Node"("FPGA I/O In"=refnum<k21> "IO Socket\\SI 1 Deserializer MFP 9 Input") -> ("I/O Item"=w988)  [unwired: 1 out]
          n453 = xnode "FPGA I/O Node"("FPGA I/O In"=refnum<k21> "IO Socket\\SI 1 Deserializer MFP 10 Input") -> ("I/O Item"=w989)  [unwired: 1 out]
        }
        frame "SI 2 Deserializer" {
          n454 = xnode "FPGA I/O Node"("FPGA I/O In"=refnum<k21> "IO Socket\\SI 2 Deserializer MFP 0 Input") -> ("I/O Item"=w1025)  [unwired: 1 out]
          n455 = xnode "FPGA I/O Node"("FPGA I/O In"=refnum<k21> "IO Socket\\SI 2 Deserializer MFP 1 Input") -> ("I/O Item"=w1024)  [unwired: 1 out]
          n456 = xnode "FPGA I/O Node"("FPGA I/O In"=refnum<k21> "IO Socket\\SI 2 Deserializer MFP 2 Input") -> ("I/O Item"=w1023)  [unwired: 1 out]
          n457 = xnode "FPGA I/O Node"("FPGA I/O In"=refnum<k21> "IO Socket\\SI 2 Deserializer MFP 3 Input") -> ("I/O Item"=w1022)  [unwired: 1 out]
          n458 = xnode "FPGA I/O Node"("FPGA I/O In"=refnum<k21> "IO Socket\\SI 2 Deserializer MFP 4 Input") -> ("I/O Item"=w1021)  [unwired: 1 out]
          n459 = xnode "FPGA I/O Node"("FPGA I/O In"=refnum<k21> "IO Socket\\SI 2 Deserializer MFP 5 Input") -> ("I/O Item"=w1020)  [unwired: 1 out]
          n460 = xnode "FPGA I/O Node"("FPGA I/O In"=refnum<k21> "IO Socket\\SI 2 Deserializer MFP 6 Input") -> ("I/O Item"=w1018)  [unwired: 1 out]
          n461 = xnode "FPGA I/O Node"("FPGA I/O In"=refnum<k21> "IO Socket\\SI 2 Deserializer MFP 7 Input") -> ("I/O Item"=w1016)  [unwired: 1 out]
          n462 = xnode "FPGA I/O Node"("FPGA I/O In"=refnum<k21> "IO Socket\\SI 2 Deserializer MFP 8 Input") -> ("I/O Item"=w1013)  [unwired: 1 out]
          n463 = xnode "FPGA I/O Node"("FPGA I/O In"=refnum<k21> "IO Socket\\SI 2 Deserializer MFP 9 Input") -> ("I/O Item"=w1011)  [unwired: 1 out]
          n464 = xnode "FPGA I/O Node"("FPGA I/O In"=refnum<k21> "IO Socket\\SI 2 Deserializer MFP 10 Input") -> ("I/O Item"=w1010)  [unwired: 1 out]
        }
        frame "SI 3 Deserializer" {
          n465 = xnode "FPGA I/O Node"("FPGA I/O In"=refnum<k21> "IO Socket\\SI 3 Deserializer MFP 0 Input") -> ("I/O Item"=w1047)  [unwired: 1 out]
          n466 = xnode "FPGA I/O Node"("FPGA I/O In"=refnum<k21> "IO Socket\\SI 3 Deserializer MFP 1 Input") -> ("I/O Item"=w1046)  [unwired: 1 out]
          n467 = xnode "FPGA I/O Node"("FPGA I/O In"=refnum<k21> "IO Socket\\SI 3 Deserializer MFP 2 Input") -> ("I/O Item"=w1045)  [unwired: 1 out]
          n468 = xnode "FPGA I/O Node"("FPGA I/O In"=refnum<k21> "IO Socket\\SI 3 Deserializer MFP 3 Input") -> ("I/O Item"=w1044)  [unwired: 1 out]
          n469 = xnode "FPGA I/O Node"("FPGA I/O In"=refnum<k21> "IO Socket\\SI 3 Deserializer MFP 4 Input") -> ("I/O Item"=w1043)  [unwired: 1 out]
          n470 = xnode "FPGA I/O Node"("FPGA I/O In"=refnum<k21> "IO Socket\\SI 3 Deserializer MFP 5 Input") -> ("I/O Item"=w1042)  [unwired: 1 out]
          n471 = xnode "FPGA I/O Node"("FPGA I/O In"=refnum<k21> "IO Socket\\SI 3 Deserializer MFP 6 Input") -> ("I/O Item"=w1040)  [unwired: 1 out]
          n472 = xnode "FPGA I/O Node"("FPGA I/O In"=refnum<k21> "IO Socket\\SI 3 Deserializer MFP 7 Input") -> ("I/O Item"=w1038)  [unwired: 1 out]
          n473 = xnode "FPGA I/O Node"("FPGA I/O In"=refnum<k21> "IO Socket\\SI 3 Deserializer MFP 8 Input") -> ("I/O Item"=w1032)  [unwired: 1 out]
          n474 = xnode "FPGA I/O Node"("FPGA I/O In"=refnum<k21> "IO Socket\\SI 3 Deserializer MFP 9 Input") -> ("I/O Item"=w1035)  [unwired: 1 out]
          n475 = xnode "FPGA I/O Node"("FPGA I/O In"=refnum<k21> "IO Socket\\SI 3 Deserializer MFP 10 Input") -> ("I/O Item"=w1034)  [unwired: 1 out]
        }
        frame "SO 0 Serializer" {
          n476 = xnode "FPGA I/O Node"("FPGA I/O In"=refnum<k21> "IO Socket\\SO 0 Serializer MFP 0 Input") -> ("I/O Item"=w1065)  [unwired: 1 out]
          n477 = xnode "FPGA I/O Node"("FPGA I/O In"=refnum<k21> "IO Socket\\SO 0 Serializer MFP 1 Input") -> ("I/O Item"=w1064)  [unwired: 1 out]
          n478 = xnode "FPGA I/O Node"("FPGA I/O In"=refnum<k21> "IO Socket\\SO 0 Serializer MFP 2 Input") -> ("I/O Item"=w1063)  [unwired: 1 out]
          n479 = xnode "FPGA I/O Node"("FPGA I/O In"=refnum<k21> "IO Socket\\SO 0 Serializer MFP 3 Input") -> ("I/O Item"=w1062)  [unwired: 1 out]
          n480 = xnode "FPGA I/O Node"("FPGA I/O In"=refnum<k21> "IO Socket\\SO 0 Serializer MFP 4 Input") -> ("I/O Item"=w1058)  [unwired: 1 out]
          n481 = xnode "FPGA I/O Node"("FPGA I/O In"=refnum<k21> "IO Socket\\SO 0 Serializer MFP 6 Input") -> ("I/O Item"=w1057)  [unwired: 1 out]
          n482 = xnode "FPGA I/O Node"("FPGA I/O In"=refnum<k21> "IO Socket\\SO 0 Serializer MFP 7 Input") -> ("I/O Item"=w1056)  [unwired: 1 out]
          n483 = xnode "FPGA I/O Node"("FPGA I/O In"=refnum<k21> "IO Socket\\SO 0 Serializer MFP 8 Input") -> ("I/O Item"=w1054)  [unwired: 1 out]
        }
        frame "SO 1 Serializer" {
          n484 = xnode "FPGA I/O Node"("FPGA I/O In"=refnum<k21> "IO Socket\\SO 1 Serializer MFP 0 Input") -> ("I/O Item"=w1081)  [unwired: 1 out]
          n485 = xnode "FPGA I/O Node"("FPGA I/O In"=refnum<k21> "IO Socket\\SO 1 Serializer MFP 1 Input") -> ("I/O Item"=w1080)  [unwired: 1 out]
          n486 = xnode "FPGA I/O Node"("FPGA I/O In"=refnum<k21> "IO Socket\\SO 1 Serializer MFP 2 Input") -> ("I/O Item"=w1079)  [unwired: 1 out]
          n487 = xnode "FPGA I/O Node"("FPGA I/O In"=refnum<k21> "IO Socket\\SO 1 Serializer MFP 3 Input") -> ("I/O Item"=w1078)  [unwired: 1 out]
          n488 = xnode "FPGA I/O Node"("FPGA I/O In"=refnum<k21> "IO Socket\\SO 1 Serializer MFP 4 Input") -> ("I/O Item"=w1074)  [unwired: 1 out]
          n489 = xnode "FPGA I/O Node"("FPGA I/O In"=refnum<k21> "IO Socket\\SO 1 Serializer MFP 6 Input") -> ("I/O Item"=w1073)  [unwired: 1 out]
          n490 = xnode "FPGA I/O Node"("FPGA I/O In"=refnum<k21> "IO Socket\\SO 1 Serializer MFP 7 Input") -> ("I/O Item"=w1072)  [unwired: 1 out]
          n491 = xnode "FPGA I/O Node"("FPGA I/O In"=refnum<k21> "IO Socket\\SO 1 Serializer MFP 8 Input") -> ("I/O Item"=w1070)  [unwired: 1 out]
        }
        frame "SO 2 Serializer" {
          n492 = xnode "FPGA I/O Node"("FPGA I/O In"=refnum<k21> "IO Socket\\SO 2 Serializer MFP 0 Input") -> ("I/O Item"=w1097)  [unwired: 1 out]
          n493 = xnode "FPGA I/O Node"("FPGA I/O In"=refnum<k21> "IO Socket\\SO 2 Serializer MFP 1 Input") -> ("I/O Item"=w1096)  [unwired: 1 out]
          n494 = xnode "FPGA I/O Node"("FPGA I/O In"=refnum<k21> "IO Socket\\SO 2 Serializer MFP 2 Input") -> ("I/O Item"=w1095)  [unwired: 1 out]
          n495 = xnode "FPGA I/O Node"("FPGA I/O In"=refnum<k21> "IO Socket\\SO 2 Serializer MFP 3 Input") -> ("I/O Item"=w1094)  [unwired: 1 out]
          n496 = xnode "FPGA I/O Node"("FPGA I/O In"=refnum<k21> "IO Socket\\SO 2 Serializer MFP 4 Input") -> ("I/O Item"=w1090)  [unwired: 1 out]
          n497 = xnode "FPGA I/O Node"("FPGA I/O In"=refnum<k21> "IO Socket\\SO 2 Serializer MFP 6 Input") -> ("I/O Item"=w1089)  [unwired: 1 out]
          n498 = xnode "FPGA I/O Node"("FPGA I/O In"=refnum<k21> "IO Socket\\SO 2 Serializer MFP 7 Input") -> ("I/O Item"=w1088)  [unwired: 1 out]
          n499 = xnode "FPGA I/O Node"("FPGA I/O In"=refnum<k21> "IO Socket\\SO 2 Serializer MFP 8 Input") -> ("I/O Item"=w1086)  [unwired: 1 out]
        }
        frame "SO 3 Serializer" {
          n500 = xnode "FPGA I/O Node"("FPGA I/O In"=refnum<k21> "IO Socket\\SO 3 Serializer MFP 0 Input") -> ("I/O Item"=w1113)  [unwired: 1 out]
          n501 = xnode "FPGA I/O Node"("FPGA I/O In"=refnum<k21> "IO Socket\\SO 3 Serializer MFP 1 Input") -> ("I/O Item"=w1112)  [unwired: 1 out]
          n502 = xnode "FPGA I/O Node"("FPGA I/O In"=refnum<k21> "IO Socket\\SO 3 Serializer MFP 2 Input") -> ("I/O Item"=w1111)  [unwired: 1 out]
          n503 = xnode "FPGA I/O Node"("FPGA I/O In"=refnum<k21> "IO Socket\\SO 3 Serializer MFP 3 Input") -> ("I/O Item"=w1110)  [unwired: 1 out]
          n504 = xnode "FPGA I/O Node"("FPGA I/O In"=refnum<k21> "IO Socket\\SO 3 Serializer MFP 4 Input") -> ("I/O Item"=w1106)  [unwired: 1 out]
          n505 = xnode "FPGA I/O Node"("FPGA I/O In"=refnum<k21> "IO Socket\\SO 3 Serializer MFP 6 Input") -> ("I/O Item"=w1105)  [unwired: 1 out]
          n506 = xnode "FPGA I/O Node"("FPGA I/O In"=refnum<k21> "IO Socket\\SO 3 Serializer MFP 7 Input") -> ("I/O Item"=w1104)  [unwired: 1 out]
          n507 = xnode "FPGA I/O Node"("FPGA I/O In"=refnum<k21> "IO Socket\\SO 3 Serializer MFP 8 Input") -> ("I/O Item"=w1102)  [unwired: 1 out]
        }
      }
      n508 = Bundle By Name(cluster=T2 {"GPIO 0"=FALSE, "GPIO 1"=FALSE, "GPIO 2"=FALSE, "GPIO 3"=FALSE, "GPIO 4"=FALSE, "GPIO 5"=FALSE, "GPIO 6"=FALSE, "GPIO 7"=FALSE, "GPIO 8"=FALSE, "GPIO 9"=FALSE, "GPIO 10"=FALSE} ("gpio bank"), "GPIO 0"=w960, "GPIO 1"=w959, "GPIO 2"=w958, "GPIO 3"=w957, "GPIO 4"=w956, "GPIO 5"=w955, "GPIO 6"=w954, "GPIO 7"=w951, "GPIO 8"=w950, "GPIO 9"=w947, "GPIO 10"=w946) -> (w953:T2)
    }
    frame condition #11 {
      n509 = case shown="\"SI 1 Deserializer\"" w1124 {
        tunnel: [_ w1153 w1175 w1193 w1209] -> w1132
        tunnel: [_ w1152 w1174 w1192 w1208] -> w1131
        tunnel: [_ w1151 w1173 w1191 w1207] -> w1130
        tunnel: [_ w1150 w1172 w1190 w1206] -> w1129
        tunnel: [_ w1149 w1171 w1186 w1202] -> w1128
        tunnel: [_ w1148 w1170 _ _] -> w1127
        tunnel: [_ w1146 w1168 w1185 w1201] -> w1126
        tunnel: [_ w1144 w1166 w1184 w1200] -> w1123
        tunnel: [_ w1141 w1163 w1182 w1198] -> w1122
        tunnel: w1121 -> [w1135 _ _ _ _]
        tunnel: [w1134 _ _ _ _] -> w1120
        tunnel: [_ w1139 w1160 _ _] -> w1119
        tunnel: [_ w1138 w1161 _ _] -> w1118
        frame Default {
          w1134 = TRUE  # serdes id invalid
          n510 = case shown="True" w1135 {
            frame False {
            }
            frame True {
              w1137 = TRUE ("enable show error")
              # "Invalid GPIO bank select"
              n511 = call <instrlib>:"Assert.vi"("assert"=w1137, "error code"=-1210, "enable show error"=w1137) -> ()  [unwired: 13 in]
            }
          }
        }
        frame "SI 0 Deserializer" {
          n512 = xnode "FPGA I/O Node"("FPGA I/O In"=refnum<k21> "IO Socket\\SI 0 Deserializer MFP 0 Input") -> ("I/O Item"=w1153)  [unwired: 1 out]
          n513 = xnode "FPGA I/O Node"("FPGA I/O In"=refnum<k21> "IO Socket\\SI 0 Deserializer MFP 1 Input") -> ("I/O Item"=w1152)  [unwired: 1 out]
          n514 = xnode "FPGA I/O Node"("FPGA I/O In"=refnum<k21> "IO Socket\\SI 0 Deserializer MFP 2 Input") -> ("I/O Item"=w1151)  [unwired: 1 out]
          n515 = xnode "FPGA I/O Node"("FPGA I/O In"=refnum<k21> "IO Socket\\SI 0 Deserializer MFP 3 Input") -> ("I/O Item"=w1150)  [unwired: 1 out]
          n516 = xnode "FPGA I/O Node"("FPGA I/O In"=refnum<k21> "IO Socket\\SI 0 Deserializer MFP 4 Input") -> ("I/O Item"=w1149)  [unwired: 1 out]
          n517 = xnode "FPGA I/O Node"("FPGA I/O In"=refnum<k21> "IO Socket\\SI 0 Deserializer MFP 5 Input") -> ("I/O Item"=w1148)  [unwired: 1 out]
          n518 = xnode "FPGA I/O Node"("FPGA I/O In"=refnum<k21> "IO Socket\\SI 0 Deserializer MFP 6 Input") -> ("I/O Item"=w1146)  [unwired: 1 out]
          n519 = xnode "FPGA I/O Node"("FPGA I/O In"=refnum<k21> "IO Socket\\SI 0 Deserializer MFP 7 Input") -> ("I/O Item"=w1144)  [unwired: 1 out]
          n520 = xnode "FPGA I/O Node"("FPGA I/O In"=refnum<k21> "IO Socket\\SI 0 Deserializer MFP 8 Input") -> ("I/O Item"=w1141)  [unwired: 1 out]
          n521 = xnode "FPGA I/O Node"("FPGA I/O In"=refnum<k21> "IO Socket\\SI 0 Deserializer MFP 9 Input") -> ("I/O Item"=w1139)  [unwired: 1 out]
          n522 = xnode "FPGA I/O Node"("FPGA I/O In"=refnum<k21> "IO Socket\\SI 0 Deserializer MFP 10 Input") -> ("I/O Item"=w1138)  [unwired: 1 out]
        }
        frame "SI 1 Deserializer" {
          n523 = xnode "FPGA I/O Node"("FPGA I/O In"=refnum<k21> "IO Socket\\SI 1 Deserializer MFP 0 Input") -> ("I/O Item"=w1175)  [unwired: 1 out]
          n524 = xnode "FPGA I/O Node"("FPGA I/O In"=refnum<k21> "IO Socket\\SI 1 Deserializer MFP 1 Input") -> ("I/O Item"=w1174)  [unwired: 1 out]
          n525 = xnode "FPGA I/O Node"("FPGA I/O In"=refnum<k21> "IO Socket\\SI 1 Deserializer MFP 2 Input") -> ("I/O Item"=w1173)  [unwired: 1 out]
          n526 = xnode "FPGA I/O Node"("FPGA I/O In"=refnum<k21> "IO Socket\\SI 1 Deserializer MFP 3 Input") -> ("I/O Item"=w1172)  [unwired: 1 out]
          n527 = xnode "FPGA I/O Node"("FPGA I/O In"=refnum<k21> "IO Socket\\SI 1 Deserializer MFP 4 Input") -> ("I/O Item"=w1171)  [unwired: 1 out]
          n528 = xnode "FPGA I/O Node"("FPGA I/O In"=refnum<k21> "IO Socket\\SI 1 Deserializer MFP 5 Input") -> ("I/O Item"=w1170)  [unwired: 1 out]
          n529 = xnode "FPGA I/O Node"("FPGA I/O In"=refnum<k21> "IO Socket\\SI 1 Deserializer MFP 6 Input") -> ("I/O Item"=w1168)  [unwired: 1 out]
          n530 = xnode "FPGA I/O Node"("FPGA I/O In"=refnum<k21> "IO Socket\\SI 1 Deserializer MFP 7 Input") -> ("I/O Item"=w1166)  [unwired: 1 out]
          n531 = xnode "FPGA I/O Node"("FPGA I/O In"=refnum<k21> "IO Socket\\SI 1 Deserializer MFP 8 Input") -> ("I/O Item"=w1163)  [unwired: 1 out]
          n532 = xnode "FPGA I/O Node"("FPGA I/O In"=refnum<k21> "IO Socket\\SI 1 Deserializer MFP 9 Input") -> ("I/O Item"=w1160)  [unwired: 1 out]
          n533 = xnode "FPGA I/O Node"("FPGA I/O In"=refnum<k21> "IO Socket\\SI 1 Deserializer MFP 10 Input") -> ("I/O Item"=w1161)  [unwired: 1 out]
        }
        frame "SO 0 Serializer" {
          n534 = xnode "FPGA I/O Node"("FPGA I/O In"=refnum<k21> "IO Socket\\SO 0 Serializer MFP 0 Input") -> ("I/O Item"=w1193)  [unwired: 1 out]
          n535 = xnode "FPGA I/O Node"("FPGA I/O In"=refnum<k21> "IO Socket\\SO 0 Serializer MFP 1 Input") -> ("I/O Item"=w1192)  [unwired: 1 out]
          n536 = xnode "FPGA I/O Node"("FPGA I/O In"=refnum<k21> "IO Socket\\SO 0 Serializer MFP 2 Input") -> ("I/O Item"=w1191)  [unwired: 1 out]
          n537 = xnode "FPGA I/O Node"("FPGA I/O In"=refnum<k21> "IO Socket\\SO 0 Serializer MFP 3 Input") -> ("I/O Item"=w1190)  [unwired: 1 out]
          n538 = xnode "FPGA I/O Node"("FPGA I/O In"=refnum<k21> "IO Socket\\SO 0 Serializer MFP 4 Input") -> ("I/O Item"=w1186)  [unwired: 1 out]
          n539 = xnode "FPGA I/O Node"("FPGA I/O In"=refnum<k21> "IO Socket\\SO 0 Serializer MFP 6 Input") -> ("I/O Item"=w1185)  [unwired: 1 out]
          n540 = xnode "FPGA I/O Node"("FPGA I/O In"=refnum<k21> "IO Socket\\SO 0 Serializer MFP 7 Input") -> ("I/O Item"=w1184)  [unwired: 1 out]
          n541 = xnode "FPGA I/O Node"("FPGA I/O In"=refnum<k21> "IO Socket\\SO 0 Serializer MFP 8 Input") -> ("I/O Item"=w1182)  [unwired: 1 out]
        }
        frame "SO 1 Serializer" {
          n542 = xnode "FPGA I/O Node"("FPGA I/O In"=refnum<k21> "IO Socket\\SO 1 Serializer MFP 0 Input") -> ("I/O Item"=w1209)  [unwired: 1 out]
          n543 = xnode "FPGA I/O Node"("FPGA I/O In"=refnum<k21> "IO Socket\\SO 1 Serializer MFP 1 Input") -> ("I/O Item"=w1208)  [unwired: 1 out]
          n544 = xnode "FPGA I/O Node"("FPGA I/O In"=refnum<k21> "IO Socket\\SO 1 Serializer MFP 2 Input") -> ("I/O Item"=w1207)  [unwired: 1 out]
          n545 = xnode "FPGA I/O Node"("FPGA I/O In"=refnum<k21> "IO Socket\\SO 1 Serializer MFP 3 Input") -> ("I/O Item"=w1206)  [unwired: 1 out]
          n546 = xnode "FPGA I/O Node"("FPGA I/O In"=refnum<k21> "IO Socket\\SO 1 Serializer MFP 4 Input") -> ("I/O Item"=w1202)  [unwired: 1 out]
          n547 = xnode "FPGA I/O Node"("FPGA I/O In"=refnum<k21> "IO Socket\\SO 1 Serializer MFP 6 Input") -> ("I/O Item"=w1201)  [unwired: 1 out]
          n548 = xnode "FPGA I/O Node"("FPGA I/O In"=refnum<k21> "IO Socket\\SO 1 Serializer MFP 7 Input") -> ("I/O Item"=w1200)  [unwired: 1 out]
          n549 = xnode "FPGA I/O Node"("FPGA I/O In"=refnum<k21> "IO Socket\\SO 1 Serializer MFP 8 Input") -> ("I/O Item"=w1198)  [unwired: 1 out]
        }
      }
      n550 = Bundle By Name(cluster=T2 {"GPIO 0"=FALSE, "GPIO 1"=FALSE, "GPIO 2"=FALSE, "GPIO 3"=FALSE, "GPIO 4"=FALSE, "GPIO 5"=FALSE, "GPIO 6"=FALSE, "GPIO 7"=FALSE, "GPIO 8"=FALSE, "GPIO 9"=FALSE, "GPIO 10"=FALSE} ("gpio bank"), "GPIO 0"=w1132, "GPIO 1"=w1131, "GPIO 2"=w1130, "GPIO 3"=w1129, "GPIO 4"=w1128, "GPIO 5"=w1127, "GPIO 6"=w1126, "GPIO 7"=w1123, "GPIO 8"=w1122, "GPIO 9"=w1119, "GPIO 10"=w1118) -> (w1125:T2)
    }
  }
  "gpio bank input" <- w5
  n551 = Not(x=w2) -> (.not. x?=→"serdes id valid":bool)
